vi "MainCondenser.vi"() -> ()   [LabVIEW 2017]
uses:
  <vilib>/Utility/miscctls.llb/LVRowAndColumnTypeDef.ctl
  <vilib>/Utility/sysdir.llb/System Directory Type.ctl
  <vilib>/Utility/config.llb/Read Key (String).vi
  <vilib>/Utility/config.llb/Write Key (String).vi
  <vilib>/Utility/cursorutil.llb/Set Cursor (Icon Pict).vi
  <vilib>/Utility/config.llb/NI_LVConfig.lvlib
panel:
  out "TesterCOM":refnum<visa-resource-name>
  out "CurrentSens":bool
  out "CurrentOut":dbl
  out "Current":string
  out "VISA Current":refnum<visa-resource-name>
  out "TestinExecution":string
  out "FullSpeed2 Current":dbl
  out "FullSpeed1 Current":dbl
  out "String":string
  out "ParamVersion":string
  out "DSP Board S/N":string
  out "POWER Board S/N":string caption="DRIVER Board S/N"
  in  "EventTimeout":i32=100
  out "TestArray":string[](array[string])
  out "Motor Speed RPM Serial":dbl
  out "PN":string
  out "FileName":string
  out "VenableSpeed":u16
  out "TesterVersion":string
  out "ClosePanel":bool=TRUE
  out "UUT SN Report":string
  out "Automation":bool
  out "Test Failed":bool
  out "VenableDirectionResult":bool
  out "VenableResult":bool
  out "ComTestResult":bool=TRUE
  out "UUT SoftwareVer":string
  out "Next SN":i32
  in  "SetSN":bool
  out "Current SN":i32
  out "FullSpeed2 Speed":dbl
  out "FullSpeed2 Current":dbl
  out "FullSpeed1 Current":dbl
  out "FullSpeed1 Speed":dbl
  out "UUT":u8
  out "Tester Status":bool
  out "UUT":string="EBAY"
  in  "Logger Path":path
  in  "Report":bool
  in  "Start":bool
  in  "ATR":string[][](table)=[["Test Communication", "-", "-", "-", "-", ""], ["Set S/N", "-", "-", "-", "-", ""], ["Set Board Number", "-", "-", "-", "-", ""], [" ", "", "", "", "", ""], ["Test Communication", "-", "-", "-", "-", ""], ["Get S/N", "-", "-", "-", "", ""], ["Get Board Number", "-", "-", "-", "", ""], ["Get FW", "-", "-", "-", "", ""], ["Enable Motor", "", "", "", "", ""], ["Small position command", "", "", "", "", ""], ["Measure delta", "", "", "", "", ""], ["Velocity command", "", "", "", "", ""]]
  in  "Settings":bool
  in  "Refresh Button":bool
  out "Serial Status":bool
  in  "VISA Kinetics":refnum<visa-resource-name>="COM6"
  in  "Serial Com":bool
  in  "Help Button":bool
  out "Pannel User Message":string
  in  "Stop Button":bool
  # "Kinetics"
  # "REDLER TECHNOLOGIES LTD"
  # "ver 1.2p"
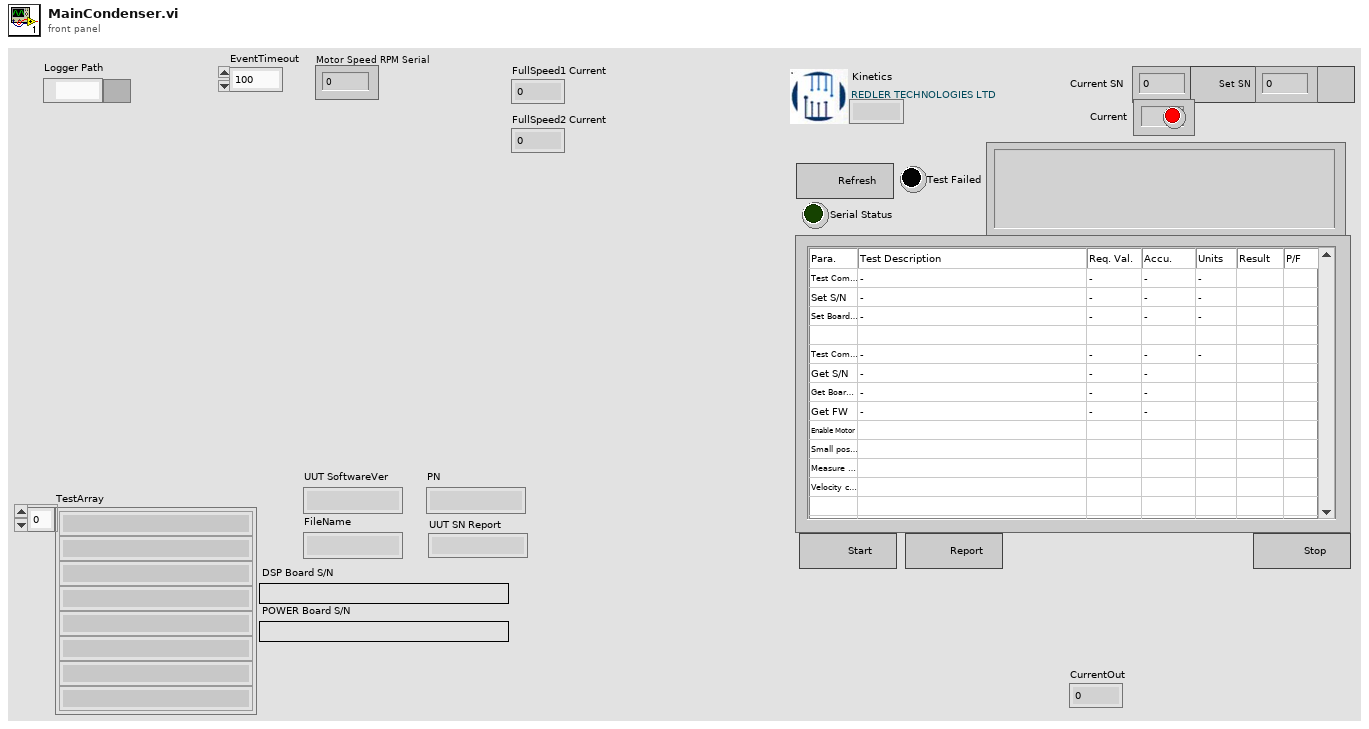
[diagram p1: front panel]
types:
  T1 = cluster{"VISA":refnum<visa-resource-name>, "TestArray":string[]}
  T2 = enum16{"Erase ATR Table", "Stop", "MainProgram", "Initialize"}
  T3 = typedef "NI_LVConfig.lvlib/Config Data RefNum.ctl" = refnum<k1>
  T4 = enum16{"Wait", "Exit", "VC=0", "ReadVC", "VC=1000"}
  T5 = enum16{"Stop", "Result", "FullSpeed2", "MD[1]=1", "FullSpeed1", "MD[1]=0"}
  T6 = enum16{"K15", "K16", "K17", "Venable", "Firmeware", "Fan", "Power", "120C", "110C", "100C", "90C", "80C", "70C", "60C", "50C", "40C", "30C", "25C", "20C", "10C", "0C"}
  T7 = enum8{"Term1", "Term2", "Current", "Fan", "TempCPU"}
  T8 = enum16{"Exit", "Wait", "ReadCurrent", "ReadTemp", "Init"}
  T9 = enum8{"Enabled", "Disabled", "Disabled and Grayed Out"}
  T10 = typedef "LVRowAndColumnTypeDef.ctl" = cluster{"Row":i32, "Column":i32}
  T11 = enum32{"Invalid", "Standard", "Closed", "Hidden", "Minimized", "Maximized"}
  T12 = enum16{"open", "replace", "create", "open or create", "replace or create", "replace or create with confirmation"}
  T13 = typedef "LVPoint32TypeDef.ctl" = cluster{"Horizontal":i32, "Vertical":i32}
  T14 = typedef "System Directory Type.ctl" = i32
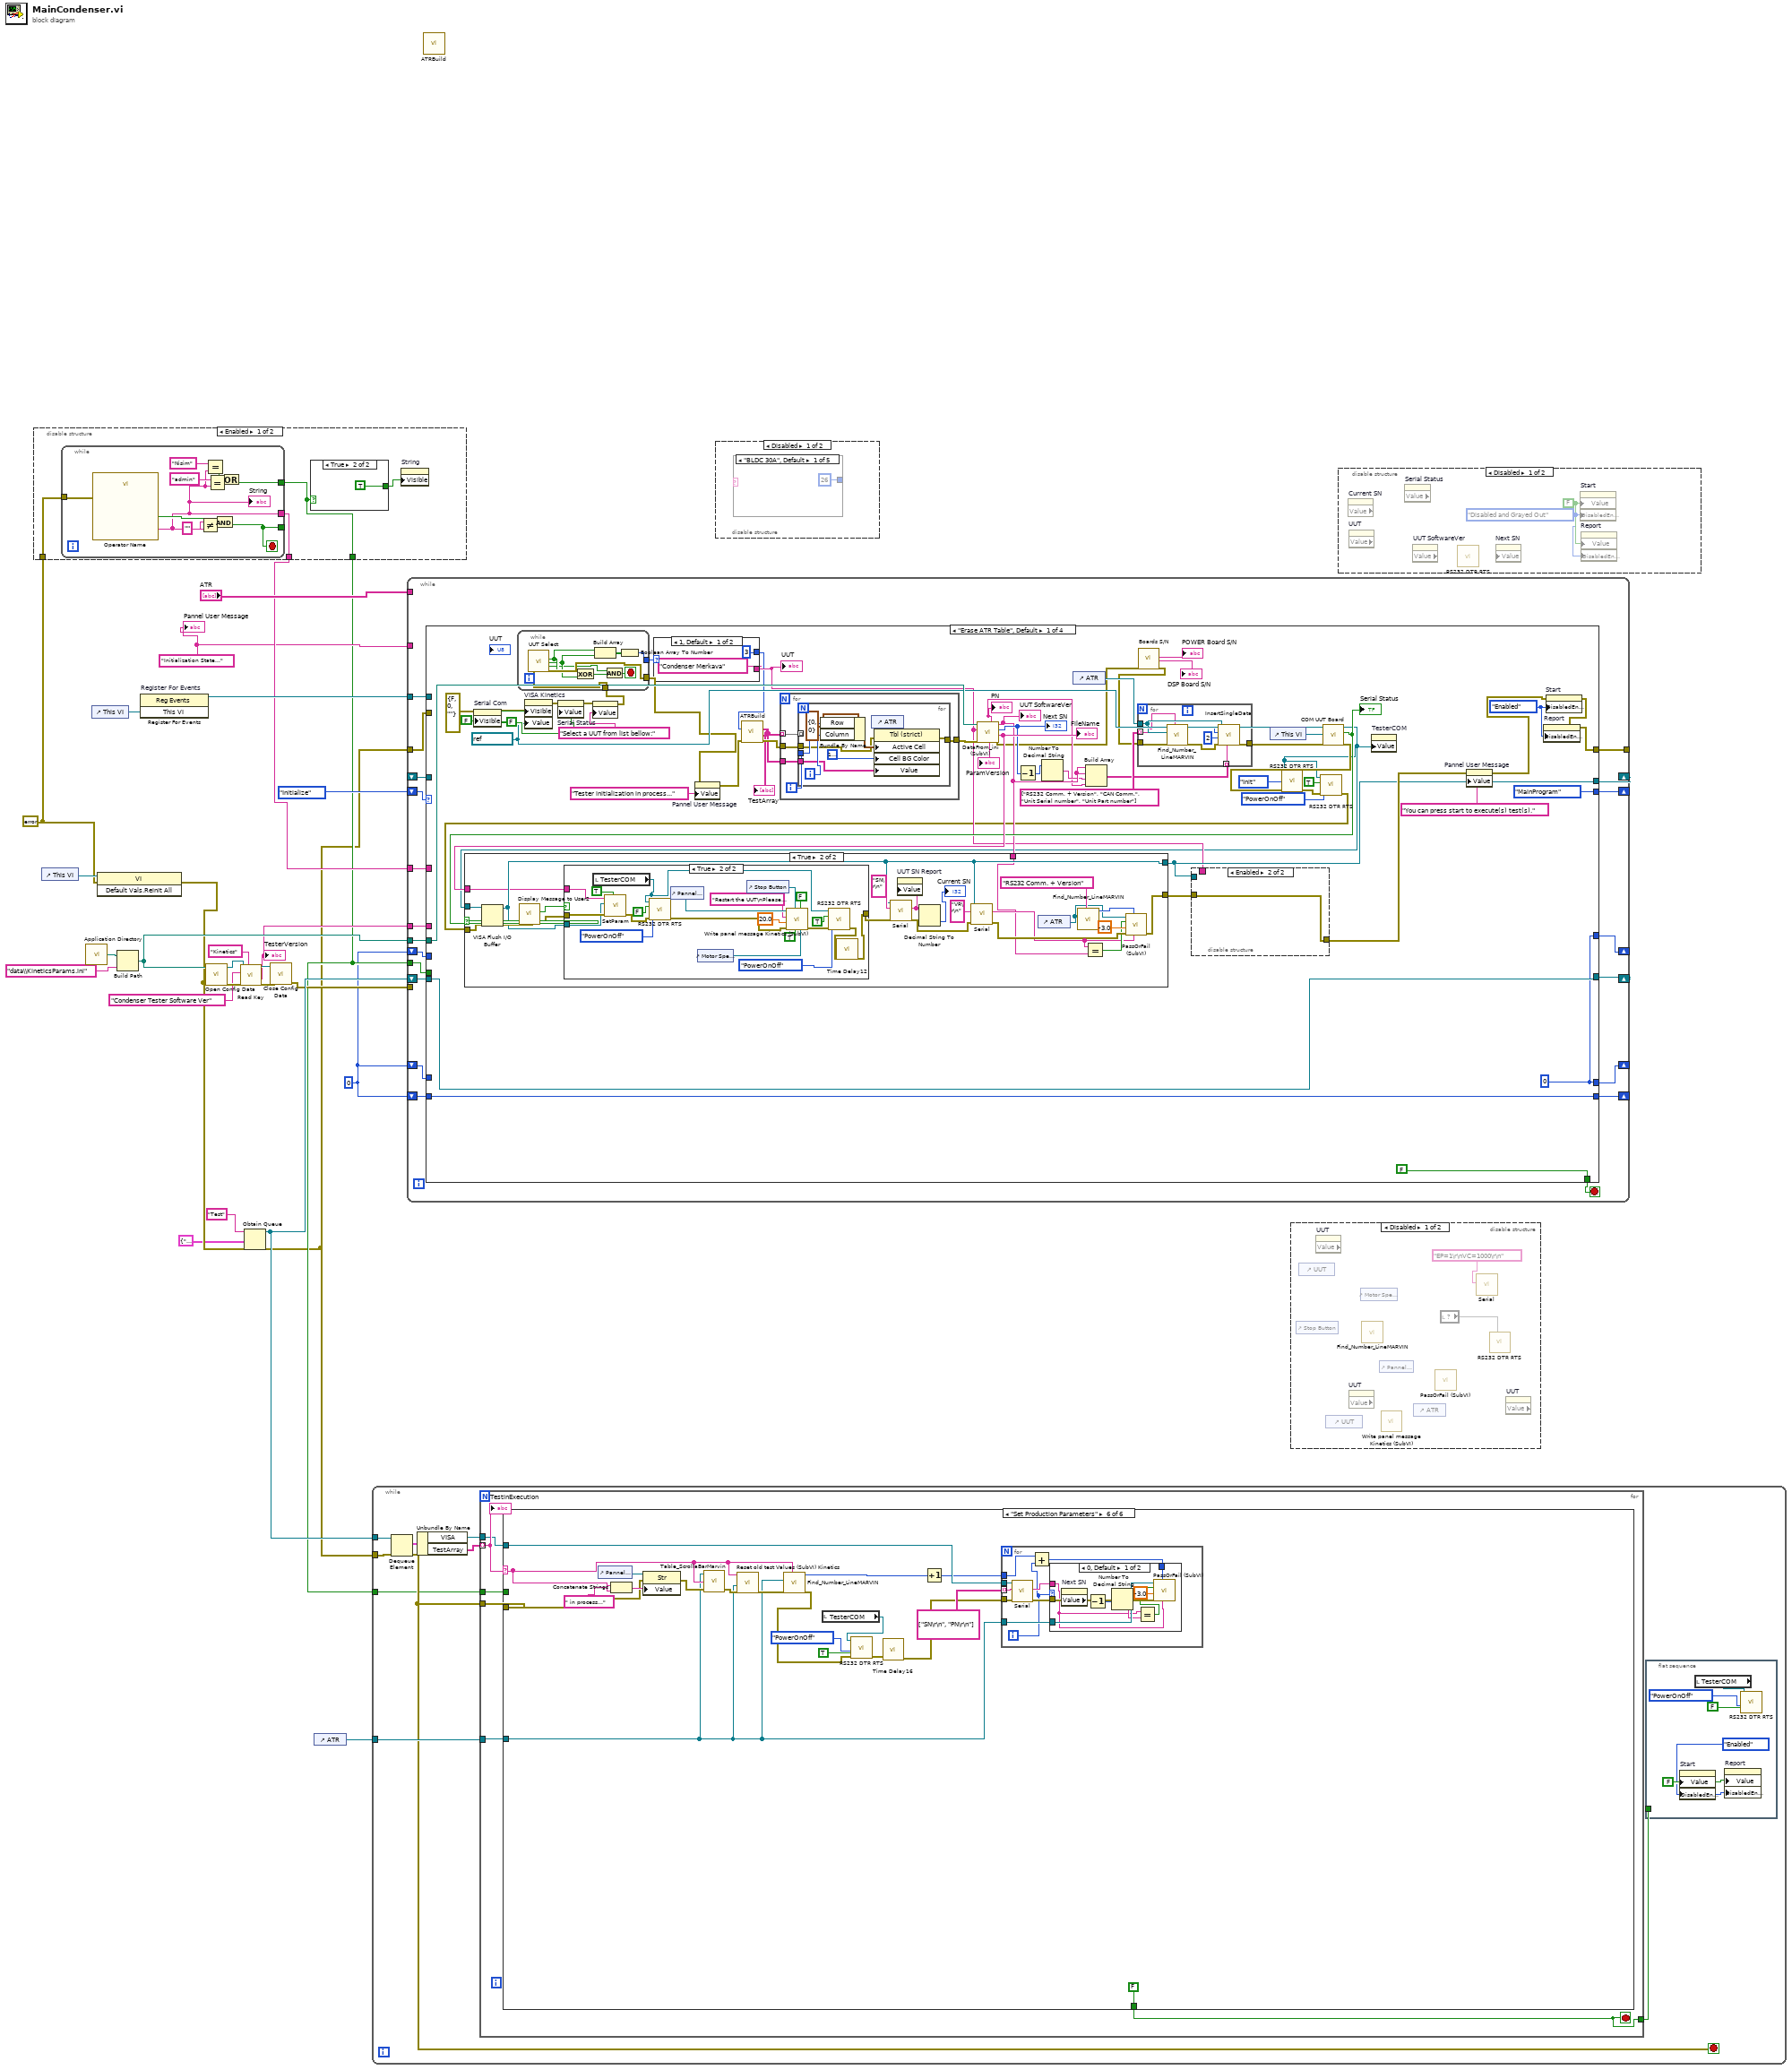
[diagram p0: block diagram]
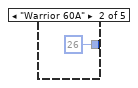
[diagram p2: hidden frame]
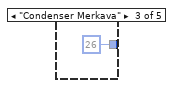
[diagram p3: hidden frame]
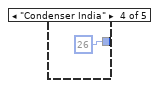
[diagram p4: hidden frame]
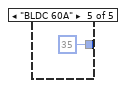
[diagram p5: hidden frame]
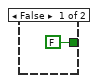
[diagram p7: hidden frame]
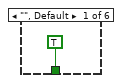
[diagram p11: hidden frame]
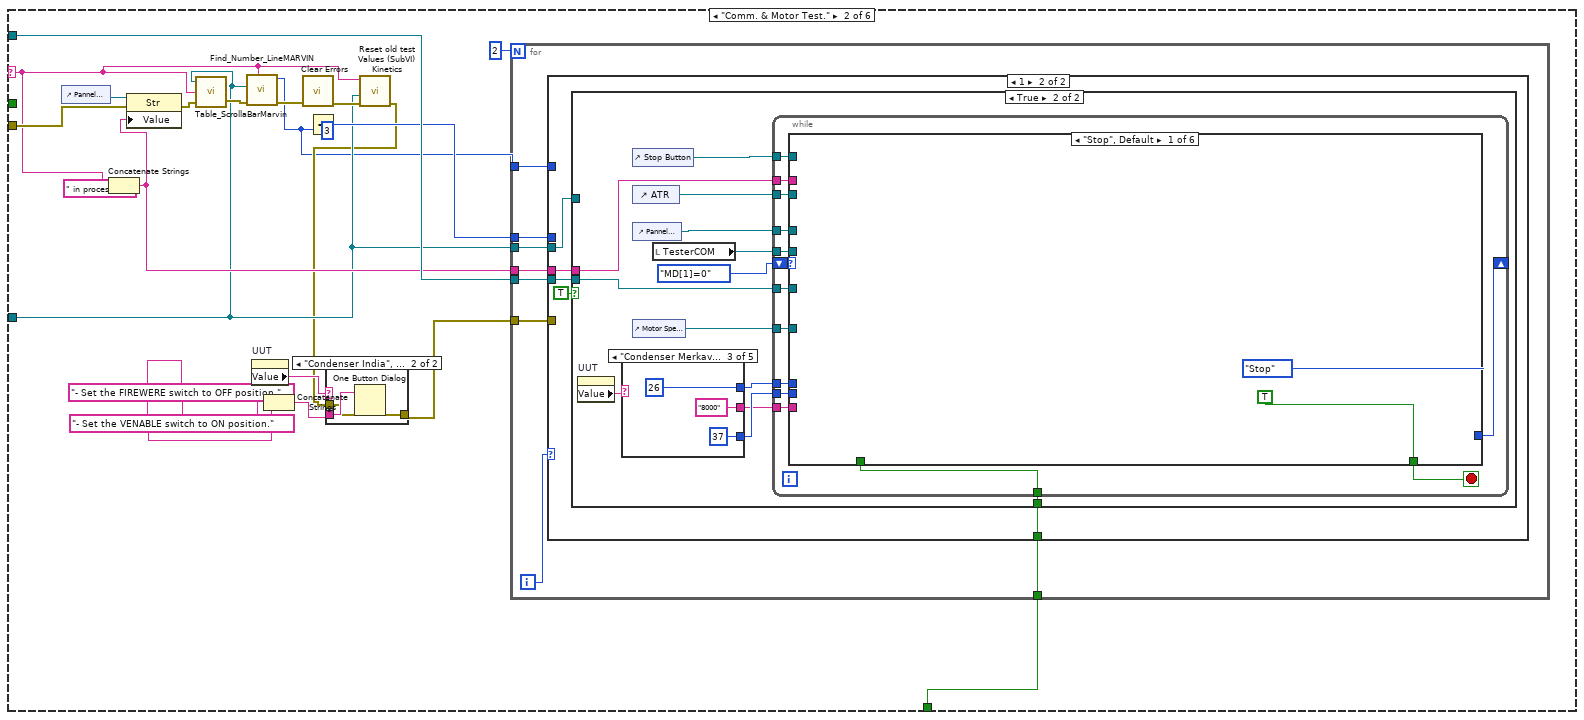
[diagram p12: hidden frame]
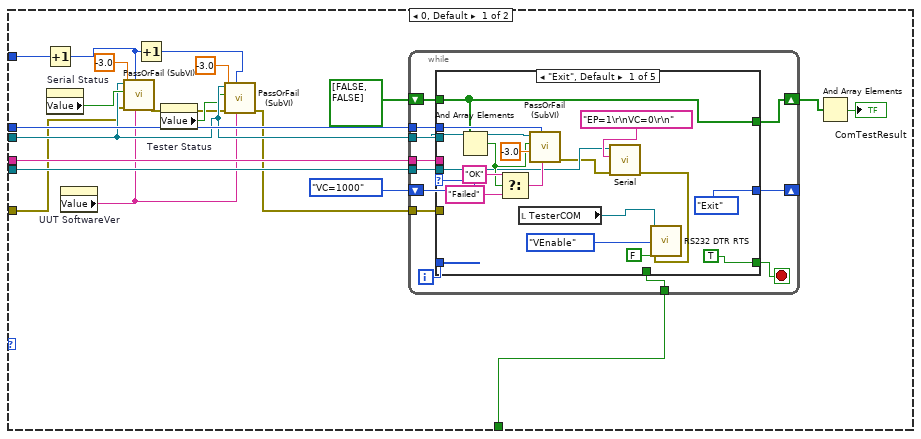
[diagram p13: hidden frame]
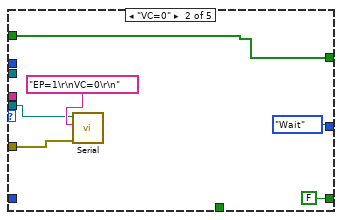
[diagram p14: hidden frame]
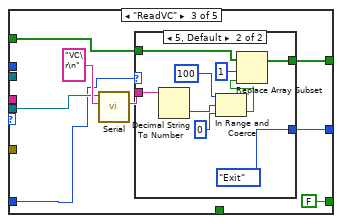
[diagram p15: hidden frame]
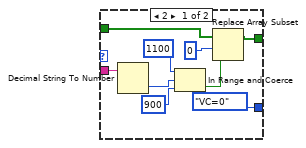
[diagram p16: hidden frame]
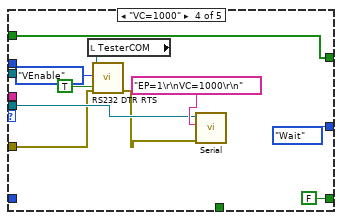
[diagram p17: hidden frame]
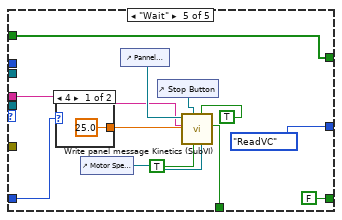
[diagram p18: hidden frame]
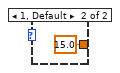
[diagram p19: hidden frame]
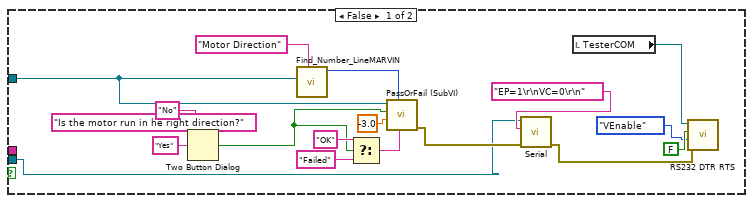
[diagram p20: hidden frame]
diagram:
  w18 = "Initialization State..."
  w3 = 0
  w6 = errorcluster {"status"=FALSE, "code"=0, "source"=""} ("error in (no error)")
  n1 = disable-structure shown="Enabled" {
    disable-tunnel: [w31 _] -> w19
    disable-tunnel: w6 -> [w29 _]
    disable-tunnel: [w28 _] -> w4
    frame Enabled {
      n2 = while {
        tunnel: [w41] -> _
        tunnel: [w34] -> w31
        tunnel: [w38] -> w28
        tunnel: w29 -> [w35]
        stop <- w41 stop-if-true
        n3 = call "Operator Name"("error in (no error)"=w35) -> ("Operator Name"=w34:string, "OK"=w42:bool)  [unwired: 16 in, 1 out]
        "String" <- w34
        n4 = Not Equal?(x=w34, y="") -> (x != y?=w43:bool)
        n5 = Equal?(x="Nisim", y=w34) -> (x = y?=w36:bool)
        n6 = Equal?(x="admin", y=w34) -> (x = y?=w39:bool)
        n7 = And(x=w42, y=w43) -> (x .and. y?=w41:bool)
        n8 = Or(x=w36, y=w39) -> (x .or. y?=w38:bool)
      }
      n9 = case shown="True" w28 {
        tunnel: [FALSE TRUE] -> w30
        frame False {
        }
        frame True {
        }
      }
      n10 = property on="String" class="Str"("Visible"=w30) -> ()  [unwired: 2 in, 2 out]
    }
    frame Disabled {
    }
  }
  n11 = control-ref of="This VI"() -> (w7:refnum<vi>)
  n12 = call <vilib>:"Application Directory.vi"() -> ("Application Directory"=w23:path)
  n13 = control-ref of="This VI"() -> (w21:refnum<vi>)
  n14 = invoke class="VI" method="Default Vals.Reinit All"(reference=w7, error in=w6) -> (error out=w5:errorcluster)  [unwired: 1 in, 2 out]
  n15 = Build Path(base path=w23, name or relative path="data\\KineticsParams.ini") -> (appended path=w10:path)
  n16 = register-events "Register For Events"(w21) -> (reference out=w20:refnum<event-registration>)  [unwired: 2 in, 1 out]
  n17 = call <vilib>:"Open Config Data.vi"("error in (no error)"=w5, "configuration file path"=w10) -> ("error out"=w16:errorcluster, "refnum"=w15:T3)  [unwired: 1 in, 7 out]
  n18 = call-poly <vilib>:"Read Key.vi"("section"="Kinetics", "error in (no error)"=w16, "key"="Condenser Tester Software Ver", "refnum"=w15) -> ("error out"=w13:errorcluster, "value"=w8:string, "refnum out"=w12:T3)  [unwired: 2 in, 3 out]
  "TesterVersion" <- w8
  n19 = Obtain Queue(name (unnamed)="Test", element data type=T1 {"VISA"="COM1", "TestArray"=[]}, error in (no error)=w5) -> (queue out=w25:refnum<queue>, error out=w1:errorcluster)  [unwired: 2 in, 1 out]
  n20 = call <vilib>:"Close Config Data.vi"("error in (no error)"=w13, "refnum"=w12) -> ("error out"=w11:errorcluster)  [unwired: 8 in, 1 out]
  n21 = control-ref of="ATR"() -> (w17:refnum<vi>)
  n22 = while {
    tunnel: w17 -> [w53]
    tunnel: w1 -> [w51]
    tunnel: w25 -> [w52]
    tunnel: w4 -> [w46]
    stop <- w48 stop-if-true
    n23 = Dequeue Element(queue=w52, error in (no error)=w51) -> (element=w50:T1, error out=w48:errorcluster)  [unwired: 1 in, 2 out]
    n24 = Unbundle By Name(w50) -> ("VISA"=w49:refnum<visa-resource-name>, "TestArray"=w45:string[])
    n25 = for {
      tunnel: w45 -> [w63] mode=indexing
      tunnel: w49 -> [w61]
      tunnel: w53 -> [w60]
      tunnel: w48 -> [w64]
      tunnel: [w59] -> w47
      tunnel: w46 -> [w62]
      stop <- w59 stop-if-true
      n26 = case shown="\"Set Production Parameters\"" w63 {
        selector: w63 -> [_ w82 w503 w964 w1087 w1211]
        tunnel: w60 -> [_ w75 _ _ w1095 w1209]
        tunnel: w64 -> [_ w85 _ _ w1100 w1213]
        tunnel: w62 -> [_ _ _ _ _ _]
        tunnel: w61 -> [_ w78 w502 w963 w1088 w1210]
        tunnel: [TRUE ("Stopped") w70 w501 w953 w1086 FALSE ("Stopped")] -> w59
        frame "", Default {
        }
        frame "Comm. & Motor Test." {
          n27 = control-ref of="Pannel User Message"() -> (w86:refnum<vi>)
          n28 = Concatenate Strings(w82, " in process..." ("string")) -> (w77:string)
          n29 = property class="Str"(reference=w86, error in=w85, "Value"=w77) -> (error out=w84:errorcluster)  [unwired: 1 out]
          n30 = call "Table_ScrollaBarMarvin.vi"("error in"=w84, "Line to focus"=w82, "reference in"=w75) -> ("error out"=w81:errorcluster)  [unwired: 2 out]
          n31 = call "Find_Number_LineMARVIN.vi"("Test Paragraph"=w82, "error in"=w81, "TableIn"=w75) -> ("error out"=w87:errorcluster, "Line number"=w66:i32)  [unwired: 2 in, 2 out]
          n32 = property on="UUT" class="Str"() -> ("Value"=w74:string)  [unwired: 2 in, 2 out]
          n33 = Concatenate Strings("- Set the FIREWERE switch to OFF position." ("Screen Line"), "- Set the VENABLE switch to ON position." ("Screen Line")) -> (w71:string)
          n34 = call <vilib>:"Clear Errors.vi"("error in (no error)"=w87) -> ("error out"=w80:errorcluster)  [unwired: 5 in, 1 out]
          n35 = Add(x=3, y=w66) -> (x+y=w76:i32)
          n36 = call "Reset old test Values (SubVI) Kinetics.vi"("error in"=w80, "Atr in"=w75, "Test Paragraph"=w82) -> ("error out"=w69:errorcluster)  [unwired: 6 in, 2 out]
          n37 = case shown="\"Condenser India\", \"Condenser Merkava\"" w74 {
            tunnel: w71 -> [_ w500]
            tunnel: w69 -> [w498 w499]
            tunnel: [w498 w499] -> w68
            frame "False", Default {
            }
            frame "Condenser India", "Condenser Merkava" {
              n38 = One Button Dialog(message=w500) -> ()  [unwired: 1 in, 1 out]
            }
          }
          n39 = for {
            N: 2 -> [_]
            tunnel: w78 -> [w95]
            tunnel: w77 -> [w94]
            tunnel: w76 -> [w93]
            tunnel: w75 -> [w92]
            tunnel: [w91] -> w70
            tunnel: w68 -> [w90]
            tunnel: w66 -> [w88]
            i -> [w89]
            n40 = case shown="1" w89 {
              tunnel: w95 -> [w113 w204]
              tunnel: w94 -> [w112 w203]
              tunnel: w93 -> [w110 _]
              tunnel: w92 -> [w103 w201]
              tunnel: [w108 w205] -> w91
              tunnel: w90 -> [w99 _]
              tunnel: w88 -> [w105 _]
              frame 0, Default {
                n41 = Increment(x=w105) -> (x+1=w98:i32)
                n42 = property on="Serial Status" class="Bool (strict)"() -> ("Value"=w107:bool)  [unwired: 2 in, 2 out]
                n43 = property on="UUT SoftwareVer" class="Str"() -> ("Value"=w96:string)  [unwired: 2 in, 2 out]
                n44 = call "PassOrFail (SubVI).vi"("String Res"=w96, "index (row)"=w98, "error in (no error)"=w99, "Data in"=-3.0, "Pass?Fail"=w107, "Table in"=w103) -> ("error out"=w101:errorcluster)  [unwired: 5 in]
                n45 = Increment(x=w98) -> (x+1=w97:i32)
                n46 = property on="Tester Status" class="Bool (strict)"() -> ("Value"=w102:bool)  [unwired: 2 in, 2 out]
                n47 = call "PassOrFail (SubVI).vi"("String Res"=w96, "index (row)"=w97, "error in (no error)"=w101, "Data in"=-3.0, "Pass?Fail"=w102, "Table in"=w103) -> ("error out"=w100:errorcluster)  [unwired: 5 in]
                n48 = while {
                  shift-right: [w124] -> _
                  shift-left: T4."VC=1000" -> [w127]
                  tunnel: w100 -> [w126]
                  tunnel: w113 -> [w125]
                  tunnel: w112 -> [w123]
                  shift-right: [w120] -> w109
                  shift-left: bool[] [FALSE, FALSE] -> [w121]
                  tunnel: w110 -> [w119]
                  tunnel: w103 -> [w118]
                  tunnel: [w116] -> w108
                  i -> [w122]
                  stop <- w117 stop-if-true
                  n49 = case shown="\"Exit\", Default" w127 {
                    tunnel: w126 -> [_ w150 _ w182 _]
                    tunnel: w125 -> [w132 w148 w157 w185 _]
                    tunnel: [T4."Exit" T4."Wait" w154 T4."Wait" T4."ReadVC"] -> w124
                    tunnel: w123 -> [_ _ _ _ w193]
                    tunnel: [TRUE FALSE FALSE FALSE FALSE] -> w117
                    tunnel: w122 -> [_ _ w155 _ w188]
                    tunnel: w121 -> [w131 w145 w153 w183 w190]
                    tunnel: [w131 w145 w152 w183 w190] -> w120
                    tunnel: w119 -> [w138 _ _ _ _]
                    tunnel: w118 -> [w140 _ _ _ _]
                    tunnel: [_ _ _ _ w187] -> w116
                    frame "Exit", Default {
                      n50 = And Array Elements(Boolean array=w131) -> (logical AND=w135:bool)
                      n51 = Select(t="OK", s=w135, f="Failed") -> (s? t:f=w139:string)
                      n52 = local read "TesterCOM"() -> (w128:refnum<visa-resource-name>)
                      n53 = call "PassOrFail (SubVI).vi"("String Res"=w139, "index (row)"=w138, "Data in"=-3.0, "Pass?Fail"=w135, "Table in"=w140) -> ("error out"=w130:errorcluster)  [unwired: 6 in]
                      n54 = call "Serial.vi"("error in (no error)"=w130, "write buffer"="EP=1\r\nVC=0\r\n", "VISA resource name"=w132) -> ("error out"=w133:errorcluster)  [unwired: 7 in, 1 out]
                      n55 = call "RS232 DTR RTS.vi"("error in (no error)"=w133, "Func"=enum16{"Init", "VEnable", "PowerOnOff"}."VEnable", "On/Off"=FALSE, "TesterCOM in"=w128) -> ()  [unwired: 7 in, 1 out]
                    }
                    frame "VC=0" {
                      n56 = call "Serial.vi"("error in (no error)"=w150, "write buffer"="EP=1\r\nVC=0\r\n", "VISA resource name"=w148) -> ()  [unwired: 7 in, 2 out]
                    }
                    frame "ReadVC" {
                      n57 = call "Serial.vi"("write buffer"="VC\r\n", "VISA resource name"=w157) -> ("read buffer"=w156:string)  [unwired: 8 in, 1 out]
                      n58 = case shown="5, Default" w155 {
                        tunnel: w156 -> [w166 w172]
                        tunnel: [T4."VC=0" T4."Exit"] -> w154
                        tunnel: w153 -> [w161 w171]
                        tunnel: [w159 w168] -> w152
                        frame 2 {
                          n59 = Decimal String To Number(string=w166) -> (number=w165:i32)  [unwired: 2 in, 1 out]
                          n60 = In Range and Coerce(upper limit=1100, x=w165, lower limit=900) -> (In Range?=w160:bool)  [unwired: 1 out]
                          n61 = Replace Array Subset(array=w161, new element=w160, index=0) -> (w159:bool[])
                        }
                        frame 5, Default {
                          n62 = Decimal String To Number(string=w172) -> (number=w175:i32)  [unwired: 2 in, 1 out]
                          n63 = In Range and Coerce(upper limit=100, x=w175, lower limit=0) -> (In Range?=w169:bool)  [unwired: 1 out]
                          n64 = Replace Array Subset(array=w171, new element=w169, index=1) -> (w168:bool[])
                        }
                      }
                    }
                    frame "VC=1000" {
                      n65 = local read "TesterCOM"() -> (w177:refnum<visa-resource-name>)
                      n66 = call "RS232 DTR RTS.vi"("error in (no error)"=w182, "Func"=enum16{"Init", "VEnable", "PowerOnOff"}."VEnable", "On/Off"=TRUE, "TesterCOM in"=w177) -> ("error out"=w181:errorcluster)  [unwired: 7 in]
                      n67 = call "Serial.vi"("error in (no error)"=w181, "write buffer"="EP=1\r\nVC=1000\r\n", "VISA resource name"=w185) -> ()  [unwired: 7 in, 2 out]
                    }
                    frame "Wait" {
                      n68 = case shown="4" w188 {
                        tunnel: [25.0 ("Time to wait") 15.0 ("Time to wait")] -> w194
                        frame 4 {
                        }
                        frame 1, Default {
                        }
                      }
                      n69 = control-ref of="Motor Speed RPM Serial"() -> (w198:refnum<vi>)
                      n70 = control-ref of="Pannel User Message"() -> (w197:refnum<vi>)
                      n71 = control-ref of="Stop Button"() -> (w192:refnum<vi>)
                      n72 = call "Write panel message Kinetics (SubVI).vi"(4:"rpm"=w198, 5:"rpm"=TRUE ("rpm"), "PrintTime"=TRUE, "Stop"=w192, "Time to wait"=w194, "Strin"=w193, "String in"=w197) -> ("Stopped"=w187:bool)  [unwired: 3 in, 1 out]
                    }
                  }
                }
                n73 = And Array Elements(Boolean array=w109) -> (logical AND=→"ComTestResult":bool)
              }
              frame 1 {
                n74 = case shown="True" TRUE {
                  tunnel: [_ w227] -> w205
                  tunnel: w204 -> [w208 w226]
                  tunnel: w203 -> [_ w224]
                  tunnel: w201 -> [w213 _]
                  frame False {
                    n75 = Two Button Dialog(message="Is the motor run in he right direction?", 1:"No" ("F button name (\"Cancel\")"), 2:"Yes" ("T button name (\"OK\")")) -> (T button?=w209:bool)
                    n76 = call "Find_Number_LineMARVIN.vi"("Test Paragraph"="Motor Direction", "TableIn"=w213) -> ("Line number"=w223:i32)  [unwired: 3 in, 3 out]
                    n77 = Select(t="OK", s=w209, f="Failed") -> (s? t:f=w222:string)
                    n78 = call "PassOrFail (SubVI).vi"("String Res"=w222, "index (row)"=w223, "Data in"=-3.0, "Pass?Fail"=w209, "Table in"=w213) -> ("error out"=w220:errorcluster)  [unwired: 6 in]
                    n79 = call "Serial.vi"("error in (no error)"=w220, "write buffer"="EP=1\r\nVC=0\r\n", "VISA resource name"=w208) -> ("error out"=w221:errorcluster)  [unwired: 7 in, 1 out]
                    n80 = local read "TesterCOM"() -> (w207:refnum<visa-resource-name>)
                    n81 = call "RS232 DTR RTS.vi"("error in (no error)"=w221, "Func"=enum16{"Init", "VEnable", "PowerOnOff"}."VEnable", "On/Off"=FALSE, "TesterCOM in"=w207) -> ()  [unwired: 7 in, 1 out]
                  }
                  frame True {
                    n82 = property on="UUT" class="Str"() -> ("Value"=w229:string)  [unwired: 2 in, 2 out]
                    n83 = case shown="\"Condenser Merkava\"" w229 {
                      tunnel: [26 26 26 26 40] -> w230
                      tunnel: [_ _ 37 37 56] -> w231
                      tunnel: [_ _ "8000" "8000" "10800"] -> w225
                      frame "BLDC 30A", Default {
                      }
                      frame "Warrior 60A" {
                      }
                      frame "Condenser Merkava" {
                      }
                      frame "Condenser India" {
                      }
                      frame "BLDC 60A" {
                      }
                    }
                    n84 = control-ref of="Stop Button"() -> (w232:refnum<vi>)
                    n85 = control-ref of="ATR"() -> (w236:refnum<vi>)
                    n86 = control-ref of="Pannel User Message"() -> (w233:refnum<vi>)
                    n87 = control-ref of="Motor Speed RPM Serial"() -> (w234:refnum<vi>)
                    n88 = local read "TesterCOM"() -> (w235:refnum<visa-resource-name>)
                    n89 = while {
                      shift-right: [w249] -> _
                      shift-left: T5."MD[1]=0" -> [w250]
                      tunnel: w232 -> [w248]
                      tunnel: w233 -> [w247]
                      tunnel: w234 -> [w246]
                      tunnel: w235 -> [w245]
                      tunnel: w230 -> [w244]
                      tunnel: w231 -> [w243]
                      tunnel: w236 -> [w242]
                      tunnel: [w237] -> w227
                      tunnel: w226 -> [w240]
                      tunnel: w225 -> [w239]
                      tunnel: w224 -> [w238]
                      stop <- w241 stop-if-true
                      n90 = case shown="\"Stop\", Default" w250 {
                        tunnel: [T5."Stop" T5."Stop" w316 w389 w413 w486] -> w249
                        tunnel: [TRUE w266 FALSE FALSE FALSE FALSE] -> w241
                        tunnel: w248 -> [_ w258 w301 w369 w399 w466]
                        tunnel: w247 -> [_ w257 w302 w370 w400 w467]
                        tunnel: w246 -> [_ w256 w303 w364 w402 w461]
                        tunnel: w245 -> [_ w254 w306 w348 _ w445]
                        tunnel: w244 -> [_ _ _ _ w401 _]
                        tunnel: w243 -> [_ _ w300 _ _ _]
                        tunnel: w242 -> [_ w268 _ _ _ _]
                        tunnel: w240 -> [_ w262 w296 w353 w397 w458]
                        tunnel: w239 -> [_ _ w295 _ w394 _]
                        tunnel: w238 -> [_ _ w293 w361 w392 w457]
                        tunnel: [_ _ w292 w354 w391 w450] -> w237
                        frame "Stop", Default {
                        }
                        frame "Result" {
                          n91 = property on="FullSpeed2 Current" class="DigNum (strict)"() -> ("Value"=w273:dbl)  [unwired: 2 in, 2 out]
                          n92 = property on="FullSpeed1 Current" class="DigNum (strict)"() -> ("Value"=w272:dbl)  [unwired: 2 in, 2 out]
                          n93 = Subtract(x=w273, y=w272) -> (x-y=w280:dbl)
                          n94 = call "Find_Number_LineMARVIN.vi"("Test Paragraph"="Motor Direction", "TableIn"=w268) -> ("Line number"=w277:i32)  [unwired: 3 in, 3 out]
                          n95 = Absolute Value(x=w280) -> (abs(x)=w275:dbl)
                          n96 = Greater Or Equal?(x=w275, y=u32 5) -> (x >= y?=w267:bool)
                          n97 = Select(t="OK", s=w267, f="Failed") -> (s? t:f=w269:string)
                          n98 = call "PassOrFail (SubVI).vi"("String Res"=w269, "index (row)"=w277, "Data in"=-3.0, "Pass?Fail"=w267, "Table in"=w268) -> ("error out"=w261:errorcluster)  [unwired: 6 in]
                          n99 = call "Serial.vi"("error in (no error)"=w261, "write buffer"="EP=1\r\nVC=0\r\n", "VISA resource name"=w262) -> ("error out"=w265:errorcluster)  [unwired: 7 in, 1 out]
                          n100 = call "RS232 DTR RTS.vi"("error in (no error)"=w265, "Func"=enum16{"Init", "VEnable", "PowerOnOff"}."VEnable", "On/Off"=FALSE, "TesterCOM in"=w254) -> ("error out"=w259:errorcluster)  [unwired: 7 in]
                          n101 = while {
                            tunnel: w259 -> [w288]
                            tunnel: w258 -> [w287]
                            tunnel: w257 -> [w286]
                            tunnel: w256 -> [w284]
                            tunnel: "Please wait untill RPM = 0." -> [w285]
                            stop <- w281 stop-if-true
                            n102 = property class="DigNum (strict)"(reference=w284) -> ("Value"=w283:dbl)  [unwired: 1 in, 2 out]
                            n103 = call "Write panel message Kinetics (SubVI).vi"(4:"rpm"=w284, 5:"rpm"=TRUE ("rpm"), "PrintTime"=FALSE, "Stop"=w287, "error in (no error)"=w288, "Time to wait"=0.2, "Strin"=w285, "String in"=w286) -> ()  [unwired: 2 in, 2 out]
                            n104 = Less Or Equal?(x=w283, y=50.0) -> (x <= y?=w281:bool)
                          }
                          n105 = Not(x=TRUE) -> (.not. x?=w266:bool)
                        }
                        frame "FullSpeed2" {
                          n106 = Search and Replace String(input string="EP=1\r\nVC=0\r\n" ("write buffer"), search string="0", replace string=w295) -> (result string=w299:string)  [unwired: 5 in, 3 out]
                          n107 = call "Serial.vi"("write buffer"=w299, "VISA resource name"=w296) -> ("error out"=w294:errorcluster)  [unwired: 8 in, 1 out]
                          n108 = Concatenate Strings(w293, "\nFull speed operation " ("string")) -> (w310:string)
                          n109 = call "Write panel message Kinetics (SubVI).vi"(4:"rpm"=w303, 5:"rpm"=TRUE ("rpm"), "PrintTime"=TRUE, "Stop"=w301, "error in (no error)"=w294, "Time to wait"=45.0, "Strin"=w310, "String in"=w302) -> ("error out"=w313:errorcluster, "Stopped"=w305:bool)  [unwired: 2 in]
                          n110 = flat-sequence {
                            tunnel: w313 -> [w320]
                            tunnel: [w320] -> w312
                            tunnel: [w319] -> w311
                            frame #0 {
                              n111 = call <vilib>:"High Resolution Relative Seconds.vi"() -> ("relative seconds"=w319:dbl)
                            }
                          }
                          n112 = while {
                            tunnel: w312 -> [_]
                            tunnel: [w342] -> _
                            tunnel: w300 -> [w346]
                            tunnel: w311 -> [w344]
                            tunnel: w310 -> [w340]
                            tunnel: w303 -> [w333]
                            tunnel: w306 -> [_]
                            tunnel: w305 -> [w337]
                            tunnel: [w325] -> w304
                            tunnel: w302 -> [w336]
                            tunnel: w301 -> [w335]
                            tunnel: [w328] -> w292
                            stop <- w347 stop-if-true
                            n113 = call <vilib>:"High Resolution Relative Seconds.vi"() -> ("relative seconds"=w345:dbl)
                            n114 = local read "CurrentOut"() -> (w327:dbl)
                            n115 = property class="DigNum (strict)"(reference=w333) -> ("Value"=w332:dbl)  [unwired: 1 in, 2 out]
                            n116 = Subtract(x=w345, y=w344) -> (x-y=w323:dbl)
                            n117 = Greater Or Equal?(x=w323, y=60.0) -> (x >= y?=w324:bool)
                            n118 = To Double Precision Float(number=w327) -> (double precision float=w326:dbl)
                            "FullSpeed2 Current" <- w326
                            n119 = Greater Or Equal?(x=w326, y=w346) -> (x >= y?=w334:bool)
                            n120 = Greater Or Equal?(x=w323, y=15.0) -> (x >= y?=w321:bool)
                            n121 = Greater Or Equal?(x=w332, y=7200.0) -> (x >= y?=w329:bool)
                            n122 = And(x=w334, y=w329) -> (x .and. y?=w330:bool)
                            n123 = call "Write panel message Kinetics (SubVI).vi"(4:"rpm"=w333, 5:"rpm"=TRUE ("rpm"), "PrintTime"=FALSE, "Stop"=w335, "Time to wait"=0.2, "Strin"=w340, "String in"=w336) -> ("error out"=w342:errorcluster, "Stopped"=w328:bool)  [unwired: 3 in]
                            n124 = Compound Arithmetic op=OR(w321, w328, w324) -> (w325:bool)
                            n125 = call "Display Message to User4"("Enable"=w321) -> ()  [unwired: 9 in, 2 out]
                            n126 = Compound Arithmetic op=OR(w321, w328, w337, w324, w330) -> (w347:bool)
                          }
                          n127 = Select(t=T5."Stop", s=w304, f=T5."Result") -> (s? t:f=w316:T5)
                        }
                        frame "MD[1]=1" {
                          n128 = call "RS232 DTR RTS.vi"("Func"=enum16{"Init", "VEnable", "PowerOnOff"}."VEnable", "On/Off"=FALSE, "TesterCOM in"=w348) -> ("error out"=w377:errorcluster)  [unwired: 8 in]
                          n129 = Concatenate Strings(w361, "\nSet Parameters MD[1]=1" ("Strin")) -> (w371:string)
                          n130 = call "Write panel message Kinetics (SubVI).vi"(4:"rpm"=w364, 5:"rpm"=FALSE ("rpm"), "PrintTime"=FALSE, "Stop"=w369, "error in (no error)"=w377, "Time to wait"=30.0, "Strin"=w371, "String in"=w370) -> ("error out"=w376:errorcluster, "Stopped"=w355:bool)  [unwired: 2 in]
                          n131 = call "Serial.vi"("error in (no error)"=w376, "write buffer"="EP=1\r\nVC=0\r\nMD[1]=1\r\n", "VISA resource name"=w353) -> ("error out"=w374:errorcluster)  [unwired: 7 in, 1 out]
                          n132 = call "RS232 DTR RTS.vi"("error in (no error)"=w374, "Func"=enum16{"Init", "VEnable", "PowerOnOff"}."PowerOnOff", "On/Off"=FALSE, "TesterCOM in"=w348) -> ("error out"=w373:errorcluster)  [unwired: 7 in]
                          n133 = call "Write panel message Kinetics (SubVI).vi"(4:"rpm"=w364, 5:"rpm"=FALSE ("rpm"), "PrintTime"=TRUE, "Stop"=w369, "error in (no error)"=w373, "Time to wait"=25.0, "Strin"=w371, "String in"=w370) -> ("error out"=w358:errorcluster, "Stopped"=w356:bool)  [unwired: 2 in]
                          n134 = call "RS232 DTR RTS.vi"("error in (no error)"=w358, "Func"=enum16{"Init", "VEnable", "PowerOnOff"}."PowerOnOff", "On/Off"=TRUE, "TesterCOM in"=w348) -> ("error out"=w359:errorcluster)  [unwired: 7 in]
                          n135 = call "RS232 DTR RTS.vi"("error in (no error)"=w359, "Func"=enum16{"Init", "VEnable", "PowerOnOff"}."VEnable", "On/Off"=TRUE, "TesterCOM in"=w348) -> ("error out"=w366:errorcluster)  [unwired: 7 in]
                          n136 = call "Write panel message Kinetics (SubVI).vi"(4:"rpm"=w364, 5:"rpm"=FALSE ("rpm"), "PrintTime"=TRUE, "Stop"=w369, "error in (no error)"=w366, "Time to wait"=3.0, "Strin"=w371, "String in"=w370) -> ("Stopped"=w357:bool)  [unwired: 2 in, 1 out]
                          n137 = Compound Arithmetic op=OR(w357, w356, w355) -> (w354:bool)
                          n138 = Compound Arithmetic op=OR(w357, w356, w355) -> (w363:bool)
                          n139 = Select(t=T5."Stop", s=w363, f=T5."FullSpeed2") -> (s? t:f=w389:T5)
                        }
                        frame "FullSpeed1" {
                          n140 = Search and Replace String(input string="EP=1\r\nVC=0\r\n" ("write buffer"), search string="0", replace string=w394) -> (result string=w393:string)  [unwired: 5 in, 3 out]
                          n141 = call "Serial.vi"("write buffer"=w393, "VISA resource name"=w397) -> ("error out"=w398:errorcluster)  [unwired: 8 in, 1 out]
                          n142 = Concatenate Strings(w392, "\nFull speed operation " ("string")) -> (w407:string)
                          n143 = call "Write panel message Kinetics (SubVI).vi"(4:"rpm"=w402, 5:"rpm"=TRUE ("rpm"), "PrintTime"=TRUE, "Stop"=w399, "error in (no error)"=w398, "Time to wait"=45.0, "Strin"=w407, "String in"=w400) -> ("error out"=w410:errorcluster, "Stopped"=w403:bool)  [unwired: 2 in]
                          n144 = flat-sequence {
                            tunnel: w410 -> [w417]
                            tunnel: [w417] -> w409
                            tunnel: [w416] -> w408
                            frame #0 {
                              n145 = call <vilib>:"High Resolution Relative Seconds.vi"() -> ("relative seconds"=w416:dbl)
                            }
                          }
                          n146 = while {
                            tunnel: w409 -> [_]
                            tunnel: [w439] -> _
                            tunnel: w401 -> [w443]
                            tunnel: w408 -> [w441]
                            tunnel: w407 -> [w437]
                            tunnel: w402 -> [w428]
                            tunnel: w403 -> [w433]
                            tunnel: [w422] -> w390
                            tunnel: w400 -> [w432]
                            tunnel: w399 -> [w431]
                            tunnel: [w424] -> w391
                            stop <- w444 stop-if-true
                            n147 = call <vilib>:"High Resolution Relative Seconds.vi"() -> ("relative seconds"=w442:dbl)
                            n148 = local read "CurrentOut"() -> (w423:dbl)
                            n149 = property class="DigNum (strict)"(reference=w428) -> ("Value"=w427:dbl)  [unwired: 1 in, 2 out]
                            n150 = Subtract(x=w442, y=w441) -> (x-y=w420:dbl)
                            n151 = Greater Or Equal?(x=w420, y=60.0) -> (x >= y?=w421:bool)
                            n152 = To Double Precision Float(number=w423) -> (double precision float=→"FullSpeed1 Current":dbl)
                            n153 = Greater Or Equal?(x=w423, y=w443) -> (x >= y?=w430:bool)
                            n154 = Greater Or Equal?(x=w420, y=15.0) -> (x >= y?=w418:bool)
                            n155 = Greater Or Equal?(x=w427, y=7800.0) -> (x >= y?=w425:bool)
                            n156 = And(x=w425, y=w430) -> (x .and. y?=w429:bool)
                            n157 = call "Write panel message Kinetics (SubVI).vi"(4:"rpm"=w428, 5:"rpm"=TRUE ("rpm"), "PrintTime"=FALSE, "Stop"=w431, "Time to wait"=0.2, "Strin"=w437, "String in"=w432) -> ("error out"=w439:errorcluster, "Stopped"=w424:bool)  [unwired: 3 in]
                            n158 = call "Display Message to User6"("Enable"=w418) -> ()  [unwired: 9 in, 2 out]
                            n159 = Compound Arithmetic op=OR(w418, w424, w421) -> (w422:bool)
                            n160 = Compound Arithmetic op=OR(w418, w424, w433, w421, w429) -> (w444:bool)
                          }
                          n161 = Select(t=T5."Stop", s=w390, f=T5."MD[1]=1") -> (s? t:f=w413:T5)
                        }
                        frame "MD[1]=0" {
                          n162 = call "RS232 DTR RTS.vi"("Func"=enum16{"Init", "VEnable", "PowerOnOff"}."VEnable", "On/Off"=FALSE, "TesterCOM in"=w445) -> ("error out"=w474:errorcluster)  [unwired: 8 in]
                          n163 = Concatenate Strings(w457, "\nSet Parameters MD[1]=0" ("Strin")) -> (w468:string)
                          n164 = call "Write panel message Kinetics (SubVI).vi"(4:"rpm"=w461, 5:"rpm"=FALSE ("rpm"), "PrintTime"=FALSE, "Stop"=w466, "error in (no error)"=w474, "Time to wait"=0.2, "Strin"=w468, "String in"=w467) -> ("error out"=w473:errorcluster, "Stopped"=w451:bool)  [unwired: 2 in]
                          n165 = call "Serial.vi"("error in (no error)"=w473, "write buffer"="EP=1\r\nVC=0\r\nMD[1]=0\r\n", "VISA resource name"=w458) -> ("error out"=w471:errorcluster)  [unwired: 7 in, 1 out]
                          n166 = call "RS232 DTR RTS.vi"("error in (no error)"=w471, "Func"=enum16{"Init", "VEnable", "PowerOnOff"}."PowerOnOff", "On/Off"=FALSE, "TesterCOM in"=w445) -> ("error out"=w470:errorcluster)  [unwired: 7 in]
                          n167 = call "Write panel message Kinetics (SubVI).vi"(4:"rpm"=w461, 5:"rpm"=FALSE ("rpm"), "PrintTime"=TRUE, "Stop"=w466, "error in (no error)"=w470, "Time to wait"=25.0, "Strin"=w468, "String in"=w467) -> ("error out"=w456:errorcluster, "Stopped"=w452:bool)  [unwired: 2 in]
                          n168 = call "RS232 DTR RTS.vi"("error in (no error)"=w456, "Func"=enum16{"Init", "VEnable", "PowerOnOff"}."PowerOnOff", "On/Off"=TRUE, "TesterCOM in"=w445) -> ("error out"=w455:errorcluster)  [unwired: 7 in]
                          n169 = call "RS232 DTR RTS.vi"("error in (no error)"=w455, "Func"=enum16{"Init", "VEnable", "PowerOnOff"}."VEnable", "On/Off"=TRUE, "TesterCOM in"=w445) -> ("error out"=w463:errorcluster)  [unwired: 7 in]
                          n170 = call "Write panel message Kinetics (SubVI).vi"(4:"rpm"=w461, 5:"rpm"=FALSE ("rpm"), "PrintTime"=TRUE, "Stop"=w466, "error in (no error)"=w463, "Time to wait"=3.0, "Strin"=w468, "String in"=w467) -> ("Stopped"=w453:bool)  [unwired: 2 in, 1 out]
                          n171 = Compound Arithmetic op=OR(w453, w452, w451) -> (w450:bool)
                          n172 = Compound Arithmetic op=OR(w453, w452, w451) -> (w460:bool)
                          n173 = Select(t=T5."Stop", s=w460, f=T5."FullSpeed1") -> (s? t:f=w486:T5)
                        }
                      }
                    }
                  }
                }
              }
            }
          }
        }
        frame "Venable Test" {
          n174 = control-ref of="Stop Button"() -> (w507:refnum<vi>)
          n175 = control-ref of="ATR"() -> (w508:refnum<vi>)
          n176 = control-ref of="Pannel User Message"() -> (w509:refnum<vi>)
          n177 = control-ref of="Motor Speed RPM Serial"() -> (w510:refnum<vi>)
          n178 = control-ref of="UUT"() -> (w511:refnum<vi>)
          n179 = Concatenate Strings(w503, " in process..." ("Strin")) -> (w504:string)
          n180 = while {
            shift-right: [w518] -> _
            shift-left: enum16{"Stop", "Direction", "Venable", "Start"}."Start" -> [w523]
            tunnel: w507 -> [w522]
            tunnel: w508 -> [w521]
            tunnel: w509 -> [w520]
            tunnel: w510 -> [w519]
            tunnel: w511 -> [w516]
            tunnel: w504 -> [w517]
            tunnel: w503 -> [w515]
            tunnel: w502 -> [w514]
            tunnel: [w512] -> w501
            stop <- w513 stop-if-true
            n181 = case shown="\"Start\"" w523 {
              tunnel: w522 -> [_ w553 w802 w850]
              tunnel: w521 -> [_ w549 w800 w843]
              tunnel: w520 -> [_ w552 w803 w856]
              tunnel: w519 -> [_ w551 w804 _]
              tunnel: w516 -> [w524 w545 w805 _]
              tunnel: [w526 FALSE FALSE FALSE] -> w513
              tunnel: [w525 w548 w801 w854] -> w518
              tunnel: w517 -> [_ w550 w799 w849]
              tunnel: w515 -> [_ _ _ w842]
              tunnel: w514 -> [_ _ _ w845]
              tunnel: [_ _ _ w837] -> w512
              frame "Stop", Default {
                n182 = disable-structure shown="Enabled" {
                  disable-tunnel: [w529 TRUE] -> w526
                  disable-tunnel: [w528 enum16{"Stop", "Direction", "Venable", "Start"}."Stop"] -> w525
                  disable-tunnel: w524 -> [w527 _]
                  frame Disabled {
                    n183 = flat-sequence {
                      tunnel: w527 -> [_]
                      tunnel: [TRUE] -> w529
                      tunnel: [enum16{"Stop", "Direction", "Venable", "Start"}."Stop"] -> w528
                      frame #0 {
                        (unwired) u16 0 ("Motor Speed RPM")
                        (unwired) TRUE ("Remote")
                        n184 = property on="VISA Kinetics" class="VISAName"() -> (error out=w533:errorcluster, "Value"=w534:refnum<visa-resource-name>)  [unwired: 2 in, 1 out]
                        n185 = call "Serial.vi"("error in (no error)"=w533, "Clear Log"=FALSE, "write buffer"="EP=1\r\nMD[1]=1\r\n", "VISA resource name"=w534) -> ("error out"=w530:errorcluster)  [unwired: 6 in, 1 out]
                        n186 = call "CANSendMessage.vi"("error in (no error)"=w530) -> ("error out"=w539:errorcluster)  [unwired: 10 in]
                        n187 = call "TesterOption (SubVI).vi"("2 Options"=FALSE, "error in (no error)"=w539, "On/Off"=FALSE, "Tester Option"=T6."Venable") -> ("error out"=w535:errorcluster)  [unwired: 6 in, 1 out]
                        n188 = call "Time Delay9"("error in (no error)"=w535) -> ()  [unwired: 10 in, 1 out]
                      }
                      frame #1 {
                      }
                    }
                  }
                  frame Enabled {
                  }
                }
              }
              frame "Direction" {
                n189 = property on="UUT" class="DigNum (strict)"() -> ("Value"=w544:u8)  [unwired: 2 in, 2 out]
                n190 = while {
                  shift-right: [w564] -> w547
                  shift-left: T5."MD[1]=0" -> [w565]
                  tunnel: w545 -> [w562]
                  tunnel: w553 -> [w561]
                  tunnel: w552 -> [w560]
                  tunnel: w551 -> [w559]
                  tunnel: w550 -> [w558]
                  tunnel: w549 -> [w557]
                  tunnel: w544 -> [w556]
                  stop <- w563 stop-if-true
                  n191 = case shown="\"MD[1]=0\"" w565 {
                    tunnel: [T5."Stop" w589 w626 w696 w724 w794] -> w564
                    tunnel: [TRUE FALSE FALSE FALSE FALSE FALSE] -> w563
                    tunnel: w562 -> [_ _ _ _ _ _]
                    tunnel: w561 -> [_ w576 w603 w666 w704 w762]
                    tunnel: w560 -> [_ _ w602 w675 w703 w772]
                    tunnel: w559 -> [_ _ w619 w664 w718 w768]
                    tunnel: w558 -> [_ _ w614 w683 w716 w780]
                    tunnel: w557 -> [_ w580 _ _ _ _]
                    tunnel: w556 -> [_ w568 w600 _ w698 _]
                    frame "Stop", Default {
                    }
                    frame "Result" {
                      n192 = property on="FullSpeed1 Current" class="DigNum (strict)"() -> ("Value"=w584:dbl)  [unwired: 2 in, 2 out]
                      n193 = property on="FullSpeed2 Current" class="DigNum (strict)"() -> ("Value"=w585:dbl)  [unwired: 2 in, 2 out]
                      n194 = property on="FullSpeed2 Speed" class="DigNum (strict)"() -> ("Value"=w587:dbl)  [unwired: 2 in, 2 out]
                      n195 = property on="FullSpeed1 Speed" class="DigNum (strict)"() -> ("Value"=w586:dbl)  [unwired: 2 in, 2 out]
                      n196 = Subtract(x=w585, y=w584) -> (x-y=w583:dbl)
                      n197 = Absolute Value(x=w583) -> (abs(x)=w572:dbl)
                      n198 = Greater Or Equal?(x=w572, y=u32 5) -> (x >= y?=w578:bool)
                      n199 = Equal?(x=w568, y=u8 95) -> (x = y?=w570:bool)
                      n200 = case shown="True" w570 {
                        tunnel: w587 -> [_ w598]
                        tunnel: w586 -> [_ w597]
                        tunnel: [TRUE w594] -> w579
                        frame False {
                        }
                        frame True {
                          n201 = Subtract(x=w598, y=w597) -> (x-y=w599:dbl)
                          n202 = Absolute Value(x=w599) -> (abs(x)=w596:dbl)
                          n203 = Greater Or Equal?(x=w596, y=500.0) -> (x >= y?=w594:bool)
                        }
                      }
                      n204 = call "Find_Number_LineMARVIN.vi"("Test Paragraph"="Motor Rotation Direction", "TableIn"=w580) -> ("Line number"=w577:i32)  [unwired: 3 in, 3 out]
                      n205 = And(x=w579, y=w578) -> (x .and. y?=w569:bool)
                      "VenableDirectionResult" <- w569
                      n206 = call "PassOrFail (SubVI).vi"("String Res"="", "index (row)"=w577, "Data in"=-3.0, "Pass?Fail"=w569, "Table in"=w580) -> ("error out"=w575:errorcluster)  [unwired: 6 in]
                      n207 = property class="Bool (strict)"(reference=w576, error in=w575) -> ("Value"=w592:bool)  [unwired: 2 out]
                      n208 = Select(t=T5."Stop", s=w592, f=T5."Stop") -> (s? t:f=w589:T5)
                    }
                    frame "FullSpeed2" {
                      (unwired) TRUE ("Remote")
                      n209 = Concatenate Strings(w614, "\nFull speed operation " ("string")) -> (w601:string)
                      n210 = call "CANSendMessage.vi"() -> ("error out"=w621:errorcluster)  [unwired: 11 in]
                      n211 = call "Write panel message Kinetics (SubVI).vi"(4:"rpm"=w619, 5:"rpm"=TRUE ("rpm"), "PrintTime"=FALSE, "Stop"=w603, "error in (no error)"=w621, "Time to wait"=0.2, "Strin"=w601, "String in"=w602) -> ("error out"=w606:errorcluster)  [unwired: 2 in, 1 out]
                      n212 = Equal?(x=w600, y=u8 95) -> (x = y?=w609:bool)
                      n213 = Select(t=u16 15100, s=w609, f=u16 12100 ("y")) -> ()  [unwired: 1 out]
                      n214 = flat-sequence {
                        tunnel: w606 -> [w631]
                        tunnel: [w631] -> w605
                        tunnel: [w630] -> w604
                        frame #0 {
                          n215 = call <vilib>:"High Resolution Relative Seconds.vi"() -> ("relative seconds"=w630:dbl)
                        }
                      }
                      n216 = Select(t=14500.0, s=w609, f=11500.0) -> (s? t:f=w608:dbl)
                      n217 = Select(t=47.0, s=w609, f=24.0) -> (s? t:f=w607:dbl)
                      n218 = while {
                        tunnel: w619 -> [w633]
                        tunnel: w605 -> [w657]
                        tunnel: [w640] -> w616
                        tunnel: w608 -> [w653]
                        tunnel: w607 -> [w652]
                        tunnel: w604 -> [w648]
                        tunnel: w603 -> [w638]
                        tunnel: w602 -> [w639]
                        tunnel: w601 -> [w636]
                        stop <- w650 stop-if-true
                        n219 = call <vilib>:"High Resolution Relative Seconds.vi"() -> ("relative seconds"=w649:dbl)
                        n220 = Subtract(x=w649, y=w648) -> (x-y=w647:dbl)
                        n221 = property class="DigNum (strict)"(reference=w633, error in=w657) -> ("Value"=w654:dbl)  [unwired: 2 out]
                        "FullSpeed2 Speed" <- w654
                        n222 = Greater Or Equal?(x=w647, y=120.0) -> (x >= y?=w645:bool)
                        n223 = Greater Or Equal?(x=w654, y=w653) -> (x >= y?=w644:bool)
                        n224 = property class="Bool (strict)"(reference=w638) -> ("Value"=w643:bool)  [unwired: 1 in, 2 out]
                        n225 = call "GetADCTester (SubVI).vi"("GetADCTester"=T7."Current", "TimeToGet"=5) -> ("error out"=w655:errorcluster, "ADCValOutput Single"=w651:dbl)  [unwired: 7 in, 1 out]
                        "FullSpeed2 Current" <- w651
                        n226 = Greater Or Equal?(x=w651, y=w652) -> (x >= y?=w641:bool)
                        n227 = And(x=w644, y=w641) -> (x .and. y?=w642:bool)
                        n228 = Compound Arithmetic op=OR(w643, w645, w642) -> (w650:bool)
                        n229 = call "Write panel message Kinetics (SubVI).vi"(4:"rpm"=w633, 5:"rpm"=TRUE ("rpm"), "PrintTime"=FALSE, "Stop"=w638, "error in (no error)"=w655, "Time to wait"=0.2, "Strin"=w636, "String in"=w639) -> ("error out"=w640:errorcluster)  [unwired: 2 in, 1 out]
                      }
                      n230 = property class="Bool (strict)"(reference=w603, error in=w616) -> ("Value"=w629:bool)  [unwired: 2 out]
                      n231 = Select(t=T5."Stop", s=w629, f=T5."Result") -> (s? t:f=w626:T5)
                    }
                    frame "MD[1]=1" {
                      (unwired) TRUE ("Remote")
                      (unwired) u16 0 ("Motor Speed RPM")
                      n232 = Concatenate Strings(w683, "\nSet Parameters MD[1]=1" ("Strin")) -> (w674:string)
                      n233 = call "TesterOption (SubVI).vi"("2 Options"=FALSE, "On/Off"=FALSE, "Tester Option"=T6."Venable") -> ("error out"=w688:errorcluster, "VISA Refnum out"=w679:refnum<visa-resource-name>)  [unwired: 7 in]
                      n234 = call "CANSendMessage.vi"("error in (no error)"=w688) -> ("error out"=w690:errorcluster)  [unwired: 10 in]
                      n235 = call "Write panel message Kinetics (SubVI).vi"(4:"rpm"=w664, 5:"rpm"=FALSE ("rpm"), "PrintTime"=TRUE, "Stop"=w666, "error in (no error)"=w690, "Time to wait"=20.0, "Strin"=w674, "String in"=w675) -> ("error out"=w663:errorcluster)  [unwired: 2 in, 1 out]
                      n236 = property on="VISA Kinetics" class="VISAName"(error in=w663) -> (error out=w689:errorcluster, "Value"=w692:refnum<visa-resource-name>)  [unwired: 1 in, 1 out]
                      n237 = call "Serial.vi"("error in (no error)"=w689, "Clear Log"=FALSE, "write buffer"="EP=1\r\nMD[1]=1\r\n", "VISA resource name"=w692) -> ("error out"=w678:errorcluster)  [unwired: 6 in, 1 out]
                      n238 = call "TesterOption (SubVI).vi"("2 Options"=FALSE, "error in (no error)"=w678, "On/Off"=FALSE, "Tester Option"=T6."Power", "VISA Refnum in"=w679) -> ("error out"=w676:errorcluster, "VISA Refnum out"=w667:refnum<visa-resource-name>)  [unwired: 5 in]
                      n239 = call "Write panel message Kinetics (SubVI).vi"(4:"rpm"=w664, 5:"rpm"=FALSE ("rpm"), "PrintTime"=TRUE, "Stop"=w666, "error in (no error)"=w676, "Time to wait"=25.0, "Strin"=w674, "String in"=w675) -> ("error out"=w668:errorcluster)  [unwired: 2 in, 1 out]
                      n240 = call "TesterOption (SubVI).vi"("2 Options"=FALSE, "error in (no error)"=w668, "On/Off"=TRUE, "Tester Option"=T6."Venable", "VISA Refnum in"=w667) -> ("error out"=w665:errorcluster)  [unwired: 5 in, 1 out]
                      n241 = call "Time Delay8"("error in (no error)"=w665) -> ("error out"=w661:errorcluster)  [unwired: 10 in]
                      n242 = property class="Bool (strict)"(reference=w666, error in=w661) -> ("Value"=w697:bool)  [unwired: 2 out]
                      n243 = Select(t=T5."Stop", s=w697, f=T5."FullSpeed2") -> (s? t:f=w696:T5)
                    }
                    frame "FullSpeed1" {
                      (unwired) TRUE ("Remote")
                      n244 = call "CANSendMessage.vi"() -> ("error out"=w719:errorcluster)  [unwired: 11 in]
                      n245 = Concatenate Strings(w716, "\nFull speed operation " ("string")) -> (w702:string)
                      n246 = call "Write panel message Kinetics (SubVI).vi"(4:"rpm"=w718, 5:"rpm"=TRUE ("rpm"), "PrintTime"=FALSE, "Stop"=w704, "error in (no error)"=w719, "Time to wait"=0.2, "Strin"=w702, "String in"=w703) -> ("error out"=w707:errorcluster)  [unwired: 2 in, 1 out]
                      n247 = Equal?(x=w698, y=u8 95) -> (x = y?=w714:bool)
                      n248 = flat-sequence {
                        tunnel: w707 -> [w729]
                        tunnel: [w729] -> w706
                        tunnel: [w728] -> w705
                        frame #0 {
                          n249 = call <vilib>:"High Resolution Relative Seconds.vi"() -> ("relative seconds"=w728:dbl)
                        }
                      }
                      n250 = Select(t=u16 15100, s=w714, f=u16 12100 ("y")) -> ()  [unwired: 1 out]
                      n251 = Select(t=13700.0, s=w714, f=11500.0) -> (s? t:f=w709:dbl)
                      n252 = Select(t=56.0, s=w714, f=33.0) -> (s? t:f=w708:dbl)
                      n253 = while {
                        tunnel: w718 -> [w731]
                        tunnel: w706 -> [w755]
                        tunnel: [w738] -> w717
                        tunnel: w709 -> [w750]
                        tunnel: w708 -> [w747]
                        tunnel: w705 -> [w745]
                        tunnel: w704 -> [w736]
                        tunnel: w703 -> [w737]
                        tunnel: w702 -> [w734]
                        stop <- w752 stop-if-true
                        n254 = property class="DigNum (strict)"(reference=w731, error in=w755) -> ("Value"=w751:dbl)  [unwired: 2 out]
                        "FullSpeed1 Speed" <- w751
                        n255 = call <vilib>:"High Resolution Relative Seconds.vi"() -> ("relative seconds"=w746:dbl)
                        n256 = Subtract(x=w746, y=w745) -> (x-y=w744:dbl)
                        n257 = Greater Or Equal?(x=w744, y=120.0) -> (x >= y?=w742:bool)
                        n258 = Greater Or Equal?(x=w751, y=w750) -> (x >= y?=w749:bool)
                        n259 = call "GetADCTester (SubVI).vi"("GetADCTester"=T7."Current", "TimeToGet"=5) -> ("error out"=w753:errorcluster, "ADCValOutput Single"=w748:dbl)  [unwired: 7 in, 1 out]
                        "FullSpeed1 Current" <- w748
                        n260 = Greater Or Equal?(x=w748, y=w747) -> (x >= y?=w739:bool)
                        n261 = And(x=w739, y=w749) -> (x .and. y?=w740:bool)
                        n262 = property class="Bool (strict)"(reference=w736) -> ("Value"=w741:bool)  [unwired: 1 in, 2 out]
                        n263 = call "Write panel message Kinetics (SubVI).vi"(4:"rpm"=w731, 5:"rpm"=TRUE ("rpm"), "PrintTime"=FALSE, "Stop"=w736, "error in (no error)"=w753, "Time to wait"=0.2, "Strin"=w734, "String in"=w737) -> ("error out"=w738:errorcluster)  [unwired: 2 in, 1 out]
                        n264 = Compound Arithmetic op=OR(w741, w740, w742) -> (w752:bool)
                      }
                      n265 = property class="Bool (strict)"(reference=w704, error in=w717) -> ("Value"=w727:bool)  [unwired: 2 out]
                      n266 = Select(t=T5."Stop", s=w727, f=T5."MD[1]=1") -> (s? t:f=w724:T5)
                    }
                    frame "MD[1]=0" {
                      (unwired) TRUE ("Remote")
                      (unwired) u16 0 ("Motor Speed RPM")
                      n267 = Concatenate Strings(w780, "\nSet Parameters MD[1]=0" ("Strin")) -> (w771:string)
                      n268 = call "TesterOption (SubVI).vi"("2 Options"=FALSE, "On/Off"=FALSE, "Tester Option"=T6."Venable") -> ("error out"=w786:errorcluster, "VISA Refnum out"=w776:refnum<visa-resource-name>)  [unwired: 7 in]
                      n269 = call "CANSendMessage.vi"("error in (no error)"=w786) -> ("error out"=w788:errorcluster)  [unwired: 10 in]
                      n270 = call "Write panel message Kinetics (SubVI).vi"(4:"rpm"=w768, 5:"rpm"=FALSE ("rpm"), "PrintTime"=FALSE, "Stop"=w762, "error in (no error)"=w788, "Time to wait"=0.2, "Strin"=w771, "String in"=w772) -> ("error out"=w783:errorcluster)  [unwired: 2 in, 1 out]
                      n271 = property on="VISA Kinetics" class="VISAName"(error in=w783) -> (error out=w787:errorcluster, "Value"=w790:refnum<visa-resource-name>)  [unwired: 1 in, 1 out]
                      n272 = call "Serial.vi"("error in (no error)"=w787, "Clear Log"=FALSE, "write buffer"="EP=1\r\nMD[1]=0\r\n", "VISA resource name"=w790) -> ("error out"=w775:errorcluster)  [unwired: 6 in, 1 out]
                      n273 = call "TesterOption (SubVI).vi"("2 Options"=FALSE, "error in (no error)"=w775, "On/Off"=FALSE, "Tester Option"=T6."Power", "VISA Refnum in"=w776) -> ("error out"=w773:errorcluster, "VISA Refnum out"=w763:refnum<visa-resource-name>)  [unwired: 5 in]
                      n274 = call "Write panel message Kinetics (SubVI).vi"(4:"rpm"=w768, 5:"rpm"=FALSE ("rpm"), "PrintTime"=TRUE, "Stop"=w762, "error in (no error)"=w773, "Time to wait"=25.0, "Strin"=w771, "String in"=w772) -> ("error out"=w764:errorcluster)  [unwired: 2 in, 1 out]
                      n275 = call "TesterOption (SubVI).vi"("2 Options"=FALSE, "error in (no error)"=w764, "On/Off"=TRUE, "Tester Option"=T6."Venable", "VISA Refnum in"=w763) -> ("error out"=w761:errorcluster)  [unwired: 5 in, 1 out]
                      n276 = call "Time Delay4"("error in (no error)"=w761) -> ("error out"=w757:errorcluster)  [unwired: 10 in]
                      n277 = property class="Bool (strict)"(reference=w762, error in=w757) -> ("Value"=w795:bool)  [unwired: 2 out]
                      n278 = Select(t=T5."Stop", s=w795, f=T5."FullSpeed1") -> (s? t:f=w794:T5)
                    }
                  }
                }
                n279 = flat-sequence {
                  tunnel: [enum16{"Stop", "Direction", "Venable", "Start"}."Stop"] -> w548
                  tunnel: w547 -> [_]
                  frame #0 {
                  }
                }
              }
              frame "Venable" {
                n280 = call "Find_Number_LineMARVIN.vi"("Test Paragraph"="Enable Test", "TableIn"=w800) -> ("Line number"=w806:i32)  [unwired: 3 in, 3 out]
                n281 = Increment(x=w806) -> (x+1=w796:i32)
                n282 = for {
                  tunnel: u16[] [5000, 0, 5000] -> [w831] mode=indexing
                  tunnel: bool[] [TRUE, FALSE, TRUE] -> [w829] mode=indexing
                  tunnel: w796 -> [w832]
                  tunnel: w805 -> [_]
                  tunnel: w804 -> [w822]
                  tunnel: w803 -> [w825]
                  tunnel: w802 -> [w824]
                  tunnel: w800 -> [w818]
                  tunnel: w799 -> [w816]
                  tunnel: [w815] -> w798 mode=indexing
                  i -> [w833]
                  (unwired) u16 5000 ("Motor Speed RPM")
                  (unwired) TRUE ("Remote")
                  w834 = 200.0 ("y")
                  n283 = call "CANSendMessage.vi"() -> ("error out"=w828:errorcluster)  [unwired: 11 in]
                  n284 = Add(x=w832, y=w833) -> (x+y=w819:i32)
                  n285 = call "TesterOption (SubVI).vi"("2 Options"=FALSE, "error in (no error)"=w828, "On/Off"=w829, "Tester Option"=T6."Venable") -> ("error out"=w827:errorcluster)  [unwired: 6 in, 1 out]
                  n286 = call "Write panel message Kinetics (SubVI).vi"(4:"rpm"=w822, 5:"rpm"=TRUE ("rpm"), "PrintTime"=TRUE, "Stop"=w824, "error in (no error)"=w827, "Time to wait"=15.0, "Strin"=w816, "String in"=w825) -> ("error out"=w826:errorcluster)  [unwired: 2 in, 1 out]
                  n287 = property class="DigNum (strict)"(reference=w822, error in=w826) -> ("Value"=w817:dbl)  [unwired: 2 out]
                  n288 = Add(x=w831, y=w834) -> (x+y=w836:dbl)
                  n289 = Subtract(x=w831, y=w834) -> (x-y=w835:dbl)
                  n290 = In Range and Coerce(upper limit=w836, x=w817, lower limit=w835) -> (In Range?=w815:bool)  [unwired: 1 out]
                  n291 = call "PassOrFail (SubVI).vi"("index (row)"=w819, "Data in"=w817, "Pass?Fail"=w815, "Table in"=w818) -> ()  [unwired: 7 in, 1 out]
                }
                n292 = property class="Bool (strict)"(reference=w802) -> ("Value"=w813:bool)  [unwired: 1 in, 2 out]
                n293 = And Array Elements(Boolean array=w798) -> (logical AND=→"VenableResult":bool)
                n294 = Select(t=enum16{"Stop", "Direction", "Venable", "Start"}."Stop", s=w813, f=enum16{"Stop", "Direction", "Venable", "Start"}."Direction") -> (s? t:f=w801:enum16{"Stop", "Direction", "Venable", "Start"})
              }
              frame "Start" {
                n295 = property class="Str"(reference=w856, "Value"=w849) -> (error out=w853:errorcluster)  [unwired: 1 in, 1 out]
                n296 = call "Find_Number_LineMARVIN.vi"("Test Paragraph"=w842, "error in"=w853, "TableIn"=w843) -> ("error out"=w844:errorcluster, "Line number"=w841:i32)  [unwired: 2 in, 2 out]
                n297 = call "Table_ScrollaBarMarvin.vi"("error in"=w844, "Line to focus"=w842, "reference in"=w843) -> ("error out"=w857:errorcluster)  [unwired: 2 out]
                n298 = call "Reset old test Values (SubVI) Kinetics.vi"("error in"=w857, "Atr in"=w843, "Test Paragraph"=w842) -> ("error out"=w838:errorcluster)  [unwired: 6 in, 2 out]
                n299 = Increment(x=w841) -> (x+1=w840:i32)
                n300 = while {
                  shift-right: [w869] -> _
                  shift-left: T4."VC=1000" -> [w872]
                  tunnel: w838 -> [w871]
                  tunnel: w845 -> [w870]
                  tunnel: w842 -> [w868]
                  shift-right: [w865] -> w848
                  shift-left: bool[] [FALSE, FALSE] -> [w866]
                  tunnel: w840 -> [w864]
                  tunnel: w843 -> [w863]
                  shift-right: [w861] -> _
                  shift-left: dbl[] [0.0, 0.0] -> [w862]
                  tunnel: [w859] -> w837
                  i -> [w867]
                  stop <- w860 stop-if-true
                  n301 = case shown="\"Exit\", Default" w872 {
                    tunnel: w871 -> [_ w890 _ w937 _]
                    tunnel: w870 -> [_ w889 w905 w940 _]
                    tunnel: [T4."Exit" T4."Wait" w902 T4."Wait" T4."ReadVC"] -> w869
                    tunnel: w868 -> [_ _ _ _ w947]
                    tunnel: [TRUE FALSE FALSE FALSE w942] -> w860
                    tunnel: w867 -> [_ _ w903 _ _]
                    tunnel: w866 -> [w874 w887 w901 w938 w944]
                    tunnel: [w874 w887 w900 w938 w944] -> w865
                    tunnel: w864 -> [w875 _ _ _ _]
                    tunnel: w863 -> [w876 _ _ _ _]
                    tunnel: w862 -> [w873 w885 w898 w933 w943]
                    tunnel: [w873 w885 w897 w933 w943] -> w861
                    tunnel: [_ _ _ _ w942] -> w859
                    frame "Exit", Default {
                      n302 = for {
                        tunnel: w876 -> [w884]
                        tunnel: w875 -> [w883]
                        tunnel: w874 -> [w882] mode=indexing
                        tunnel: w873 -> [w879] mode=indexing
                        i -> [w880]
                        n303 = Add(x=w880, y=w883) -> (x+y=w881:i32)
                        n304 = call "PassOrFail (SubVI).vi"("index (row)"=w881, "Data in"=w879, "Pass?Fail"=w882, "Table in"=w884) -> ()  [unwired: 7 in, 1 out]
                      }
                    }
                    frame "VC=0" {
                      n305 = disable-structure shown="Enabled" {
                        disable-tunnel: w890 -> [w893 _]
                        disable-tunnel: w889 -> [w891 _]
                        frame Disabled {
                          n306 = call "Serial.vi"("error in (no error)"=w893, "write buffer"="EP=1\r\nVC=0\r\n", "VISA resource name"=w891) -> ()  [unwired: 7 in, 2 out]
                        }
                        frame Enabled {
                          n307 = local read "TesterCOM"() -> (w895:refnum<visa-resource-name>)
                          n308 = call "RS232 DTR RTS.vi"("Func"=enum16{"Init", "VEnable", "PowerOnOff"}."VEnable", "On/Off"=FALSE, "TesterCOM in"=w895) -> ()  [unwired: 8 in, 1 out]
                        }
                      }
                    }
                    frame "ReadVC" {
                      n309 = call "Serial.vi"("write buffer"="VC\r\n", "VISA resource name"=w905) -> ("read buffer"=w904:string)  [unwired: 8 in, 1 out]
                      n310 = case shown="2" w903 {
                        tunnel: w904 -> [w917 w927]
                        tunnel: [T4."VC=0" T4."Exit"] -> w902
                        tunnel: w901 -> [w913 w926]
                        tunnel: [w911 w923] -> w900
                        tunnel: w898 -> [w910 w922]
                        tunnel: [w907 w919] -> w897
                        frame 2 {
                          n311 = Decimal String To Number(string=w917) -> (number=w908:i32)  [unwired: 2 in, 1 out]
                          n312 = In Range and Coerce(upper limit=1100, x=w908, lower limit=900) -> (In Range?=w912:bool)  [unwired: 1 out]
                          n313 = Replace Array Subset(array=w910, new element=w908, index=0) -> (w907:dbl[])
                          n314 = Replace Array Subset(array=w913, new element=w912, index=0) -> (w911:bool[])
                        }
                        frame 5, Default {
                          n315 = Decimal String To Number(string=w927) -> (number=w920:i32)  [unwired: 2 in, 1 out]
                          n316 = In Range and Coerce(upper limit=100, x=w920, lower limit=0) -> (In Range?=w924:bool)  [unwired: 1 out]
                          n317 = Replace Array Subset(array=w922, new element=w920, index=1) -> (w919:dbl[])
                          n318 = Replace Array Subset(array=w926, new element=w924, index=1) -> (w923:bool[])
                        }
                      }
                    }
                    frame "VC=1000" {
                      n319 = local read "TesterCOM"() -> (w932:refnum<visa-resource-name>)
                      n320 = call "RS232 DTR RTS.vi"("error in (no error)"=w937, "Func"=enum16{"Init", "VEnable", "PowerOnOff"}."VEnable", "On/Off"=TRUE, "TesterCOM in"=w932) -> ("error out"=w936:errorcluster)  [unwired: 7 in]
                      n321 = call "Serial.vi"("error in (no error)"=w936, "write buffer"="EP=1\r\nVC=1000\r\n", "VISA resource name"=w940) -> ()  [unwired: 7 in, 2 out]
                    }
                    frame "Wait" {
                      n322 = control-ref of="Motor Speed RPM Serial"() -> (w952:refnum<vi>)
                      n323 = control-ref of="Pannel User Message"() -> (w951:refnum<vi>)
                      n324 = control-ref of="Stop Button"() -> (w946:refnum<vi>)
                      n325 = call "Write panel message Kinetics (SubVI).vi"(4:"rpm"=w952, 5:"rpm"=TRUE ("rpm"), "PrintTime"=TRUE, "Stop"=w946, "Time to wait"=20.0, "Strin"=w947, "String in"=w951) -> ("Stopped"=w942:bool)  [unwired: 3 in, 1 out]
                    }
                  }
                }
                n326 = And Array Elements(Boolean array=w848) -> ()  [unwired: 1 out]
                n327 = property class="Bool (strict)"(reference=w850) -> ("Value"=w858:bool)  [unwired: 1 in, 2 out]
                n328 = Select(t=enum16{"Stop", "Direction", "Venable", "Start"}."Stop", s=w858, f=enum16{"Stop", "Direction", "Venable", "Start"}."Stop") -> (s? t:f=w854:enum16{"Stop", "Direction", "Venable", "Start"})
              }
            }
          }
        }
        frame "Motor Thermistor Test" {
          n329 = Concatenate Strings(w964, " in process..." ("Strin")) -> (w965:string)
          n330 = control-ref of="ATR"() -> (w967:refnum<vi>)
          n331 = control-ref of="Pannel User Message"() -> (w968:refnum<vi>)
          n332 = property class="Str"(reference=w968, "Value"=w965) -> (error out=w961:errorcluster)  [unwired: 1 in, 1 out]
          n333 = call "Find_Number_LineMARVIN.vi"("Test Paragraph"=w964, "error in"=w961, "TableIn"=w967) -> ("error out"=w958:errorcluster, "Line number"=w957:i32)  [unwired: 2 in, 2 out]
          n334 = call "Table_ScrollaBarMarvin.vi"("error in"=w958, "Line to focus"=w964, "reference in"=w967) -> ("error out"=w962:errorcluster)  [unwired: 2 out]
          n335 = call "Reset old test Values (SubVI) Kinetics.vi"("error in"=w962, "Atr in"=w967, "Test Paragraph"=w964) -> ("error out"=w954:errorcluster)  [unwired: 6 in, 2 out]
          n336 = Increment(x=w957) -> (x+1=w956:i32)
          n337 = while {
            shift-right: [w979] -> _
            shift-left: T4."VC=1000" -> [w982]
            tunnel: w954 -> [w981]
            tunnel: w963 -> [w980]
            tunnel: w964 -> [w978]
            shift-right: [w974] -> _
            shift-left: bool[] [FALSE, FALSE] -> [w975]
            tunnel: w956 -> [w973]
            tunnel: w967 -> [w972]
            shift-right: [w970] -> _
            shift-left: dbl[] [0.0, 0.0] -> [w971]
            tunnel: [w969] -> w953
            i -> [w976]
            stop <- w977 stop-if-true
            n338 = case shown="\"Exit\", Default" w982 {
              tunnel: w981 -> [_ w1007 _ w1068 _]
              tunnel: w980 -> [w986 w1006 w1026 w1071 _]
              tunnel: [T4."Exit" T4."Wait" w1023 T4."Wait" T4."ReadVC"] -> w979
              tunnel: w978 -> [_ _ _ _ w1078]
              tunnel: [TRUE FALSE FALSE FALSE w1073] -> w977
              tunnel: w976 -> [_ w1001 w1024 _ _]
              tunnel: w975 -> [w990 w1004 w1022 w1069 w1075]
              tunnel: [w990 w1004 w1021 w1069 w1075] -> w974
              tunnel: w973 -> [w991 _ _ _ _]
              tunnel: w972 -> [w992 _ _ _ _]
              tunnel: w971 -> [w989 w1002 w1019 w1064 w1074]
              tunnel: [w989 w1002 w1018 w1064 w1074] -> w970
              tunnel: [_ _ _ _ w1073] -> w969
              frame "Exit", Default {
                n339 = for {
                  tunnel: w992 -> [w1000]
                  tunnel: w991 -> [w999]
                  tunnel: w990 -> [w998] mode=indexing
                  tunnel: w989 -> [w995] mode=indexing
                  i -> [w996]
                  n340 = Add(x=w996, y=w999) -> (x+y=w997:i32)
                  n341 = call "PassOrFail (SubVI).vi"("index (row)"=w997, "Data in"=w995, "Pass?Fail"=w998, "Table in"=w1000) -> ()  [unwired: 7 in, 1 out]
                }
                n342 = local read "TesterCOM"() -> (w985:refnum<visa-resource-name>)
                n343 = call "Serial.vi"("write buffer"="EP=1\r\nVC=0\r\n", "VISA resource name"=w986) -> ("error out"=w983:errorcluster)  [unwired: 8 in, 1 out]
                n344 = call "RS232 DTR RTS.vi"("error in (no error)"=w983, "Func"=enum16{"Init", "VEnable", "PowerOnOff"}."VEnable", "On/Off"=FALSE, "TesterCOM in"=w985) -> ()  [unwired: 7 in, 1 out]
              }
              frame "VC=0" {
                n345 = disable-structure shown="Enabled" {
                  disable-tunnel: w1007 -> [_ _]
                  disable-tunnel: w1006 -> [_ _]
                  disable-tunnel: w1001 -> [w1008 w1014]
                  frame Enabled {
                    n346 = case shown="6, Default" w1008 {
                      tunnel: [TRUE ("On/Off") FALSE ("On/Off")] -> w1009
                      frame 6, Default {
                      }
                      frame 3 {
                      }
                    }
                    n347 = local read "TesterCOM"() -> (w1011:refnum<visa-resource-name>)
                    n348 = call "RS232 DTR RTS.vi"("Func"=enum16{"Init", "VEnable", "PowerOnOff"}."VEnable", "On/Off"=w1009, "TesterCOM in"=w1011) -> ()  [unwired: 8 in, 1 out]
                  }
                  frame Disabled {
                    n349 = case shown="3" w1014 {
                      tunnel: ["Connect wires of the thermistor" ("message") "Disconnect wires of the thermistor" ("message")] -> w1015
                      frame 6, Default {
                      }
                      frame 3 {
                      }
                    }
                    n350 = One Button Dialog(message=w1015) -> ()  [unwired: 1 in, 1 out]
                  }
                }
              }
              frame "ReadVC" {
                n351 = call "Serial.vi"("write buffer"="VC\r\n", "VISA resource name"=w1026) -> ("read buffer"=w1025:string)  [unwired: 8 in, 1 out]
                n352 = case shown="8" w1024 {
                  tunnel: w1025 -> [w1037 w1046 w1058]
                  tunnel: [w1031 T4."VC=0" T4."Exit"] -> w1023
                  tunnel: w1022 -> [w1028 w1045 w1057]
                  tunnel: [w1028 w1042 w1054] -> w1021
                  tunnel: w1019 -> [w1029 w1041 w1053]
                  tunnel: [w1029 w1038 w1050] -> w1018
                  frame 2 {
                    n353 = Decimal String To Number(string=w1037) -> (number=w1034:i32)  [unwired: 2 in, 1 out]
                    n354 = In Range and Coerce(upper limit=1100, x=w1034, lower limit=900) -> (In Range?=w1033:bool)  [unwired: 1 out]
                    n355 = Select(t=T4."VC=0", s=w1033, f=T4."Exit") -> (s? t:f=w1031:T4)
                  }
                  frame 5, Default {
                    n356 = Decimal String To Number(string=w1046) -> (number=w1039:i32)  [unwired: 2 in, 1 out]
                    n357 = In Range and Coerce(upper limit=100, x=w1039, lower limit=0) -> (In Range?=w1043:bool)  [unwired: 1 out]
                    n358 = Replace Array Subset(array=w1041, new element=w1039, index=0) -> (w1038:dbl[])
                    n359 = Replace Array Subset(array=w1045, new element=w1043, index=0) -> (w1042:bool[])
                  }
                  frame 8 {
                    n360 = Decimal String To Number(string=w1058) -> (number=w1051:i32)  [unwired: 2 in, 1 out]
                    n361 = In Range and Coerce(upper limit=1100, x=w1051, lower limit=900) -> (In Range?=w1055:bool)  [unwired: 1 out]
                    n362 = Replace Array Subset(array=w1053, new element=w1051, index=1) -> (w1050:dbl[])
                    n363 = Replace Array Subset(array=w1057, new element=w1055, index=1) -> (w1054:bool[])
                  }
                }
              }
              frame "VC=1000" {
                n364 = local read "TesterCOM"() -> (w1063:refnum<visa-resource-name>)
                n365 = call "RS232 DTR RTS.vi"("error in (no error)"=w1068, "Func"=enum16{"Init", "VEnable", "PowerOnOff"}."VEnable", "On/Off"=TRUE, "TesterCOM in"=w1063) -> ("error out"=w1067:errorcluster)  [unwired: 7 in]
                n366 = call "Serial.vi"("error in (no error)"=w1067, "write buffer"="EP=1\r\nVC=1000\r\n", "VISA resource name"=w1071) -> ()  [unwired: 7 in, 2 out]
              }
              frame "Wait" {
                n367 = control-ref of="Motor Speed RPM Serial"() -> (w1083:refnum<vi>)
                n368 = control-ref of="Pannel User Message"() -> (w1082:refnum<vi>)
                n369 = control-ref of="Stop Button"() -> (w1077:refnum<vi>)
                n370 = call "Write panel message Kinetics (SubVI).vi"(4:"rpm"=w1083, 5:"rpm"=TRUE ("rpm"), "PrintTime"=TRUE, "Stop"=w1077, "Time to wait"=20.0, "Strin"=w1078, "String in"=w1082) -> ("Stopped"=w1073:bool)  [unwired: 3 in, 1 out]
              }
            }
          }
        }
        frame "Motor Run Test" {
          n371 = control-ref of="Pannel User Message"() -> (w1103:refnum<vi>)
          n372 = Concatenate Strings(w1087, " in process..." ("Strin")) -> (w1092:string)
          n373 = property class="Str"(reference=w1103, error in=w1100, "Value"=w1092) -> (error out=w1102:errorcluster)  [unwired: 1 out]
          n374 = call "Table_ScrollaBarMarvin.vi"("error in"=w1102, "Line to focus"=w1087, "reference in"=w1095) -> ()  [unwired: 3 out]
          n375 = call "Reset old test Values (SubVI) Kinetics.vi"("Atr in"=w1095, "Test Paragraph"=w1087) -> ("error out"=w1101:errorcluster)  [unwired: 7 in, 2 out]
          n376 = call "Find_Number_LineMARVIN.vi"("Test Paragraph"=w1087, "error in"=w1101, "TableIn"=w1095) -> ("error out"=w1098:errorcluster, "Line number"=w1094:i32)  [unwired: 2 in, 2 out]
          n377 = Increment(x=w1094) -> (x+1=w1093:i32)
          n378 = while {
            tunnel: w1098 -> [w1106]
            tunnel: w1088 -> [w1113]
            shift-right: [w1111] -> _
            shift-left: T8."Init" -> [w1112]
            tunnel: w1095 -> [w1110]
            tunnel: w1093 -> [w1109]
            tunnel: w1092 -> [w1107]
            tunnel: [w1106] -> w1089
            tunnel: [w1104] -> w1086
            i -> [w1108]
            stop <- w1105 stop-if-true
            n379 = case shown="\"Exit\", Default" w1112 {
              tunnel: w1106 -> [_ w1119 w1140 w1177 w1195]
              tunnel: w1113 -> [_ _ _ w1178 _]
              tunnel: [T8."Exit" T8."ReadTemp" w1137 T8."ReadCurrent" T8."ReadTemp"] -> w1111
              tunnel: w1110 -> [_ _ w1151 w1172 _]
              tunnel: w1109 -> [_ _ w1153 w1174 _]
              tunnel: w1108 -> [_ _ w1154 w1175 _]
              tunnel: w1107 -> [_ w1120 w1139 _ _]
              tunnel: [TRUE ("Stopped") w1117 w1133 _ _] -> w1105
              tunnel: [_ w1117 _ _ _] -> w1104
              frame "Exit", Default {
              }
              frame "Wait" {
                n380 = control-ref of="Motor Speed RPM Serial"() -> (w1125:refnum<vi>)
                n381 = control-ref of="Pannel User Message"() -> (w1124:refnum<vi>)
                n382 = control-ref of="Stop Button"() -> (w1123:refnum<vi>)
                n383 = call "Write panel message Kinetics (SubVI).vi"(4:"rpm"=w1125, 5:"rpm"=TRUE ("rpm"), "PrintTime"=TRUE, "Stop"=w1123, "error in (no error)"=w1119, "Time to wait"=1140.0, "Strin"=w1120, "String in"=w1124) -> ("Stopped"=w1117:bool)  [unwired: 2 in, 1 out]
              }
              frame "ReadCurrent" {
                w1149 = 3.0 ("x")
                n384 = control-ref of="Motor Speed RPM Serial"() -> (w1146:refnum<vi>)
                n385 = control-ref of="Pannel User Message"() -> (w1145:refnum<vi>)
                n386 = control-ref of="Stop Button"() -> (w1144:refnum<vi>)
                n387 = call "Write panel message Kinetics (SubVI).vi"(4:"rpm"=w1146, 5:"rpm"=TRUE ("rpm"), "PrintTime"=TRUE, "Stop"=w1144, "error in (no error)"=w1140, "Time to wait"=59.0, "Strin"=w1139, "String in"=w1145) -> ("error out"=w1136:errorcluster, "Stopped"=w1138:bool)  [unwired: 2 in]
                n388 = property on="UUT" class="Str"() -> ("Value"=w1135:string)  [unwired: 2 in, 2 out]
                n389 = case shown="\"True\", Default" w1135 {
                  tunnel: [w1155 w1157] -> w1134
                  tunnel: w1136 -> [_ _]
                  frame "Condenser India", "Condenser Merkava" {
                    n390 = call "Current prob"() -> ("Current"=w1155:dbl)  [unwired: 17 in, 2 out]
                  }
                  frame "True", Default {
                    n391 = local read "CurrentOut"() -> (w1156:dbl)
                    n392 = To Double Precision Float(number=w1156) -> (double precision float=w1157:dbl)
                  }
                }
                n393 = case shown="2, Default" w1154 {
                  tunnel: w1153 -> [w1160 w1163]
                  tunnel: [w1159 w1164] -> w1152
                  tunnel: [T8."Wait" T8."Exit"] -> w1137
                  frame 2, Default {
                    n394 = Increment(x=w1160) -> (x+1=w1159:i32)
                  }
                  frame 5 {
                    n395 = Add(x=w1163, y=3) -> (x+y=w1164:i32)
                  }
                }
                n396 = call "ValFromATR(SubVI).vi"("Row"=w1152, "Table in"=w1151) -> ("Val"=w1150:dbl)  [unwired: 8 in, 1 out]
                n397 = Add(x=w1149, y=w1150) -> (x+y=w1148:dbl)
                n398 = Subtract(x=w1150, y=w1149) -> (x-y=w1147:dbl)
                n399 = local read "TesterCOM"() -> (w1127:refnum<visa-resource-name>)
                n400 = In Range and Coerce(upper limit=w1148, x=w1134, lower limit=w1147) -> (In Range?=w1130:bool)  [unwired: 1 out]
                n401 = Not(x=w1130) -> (.not. x?=w1132:bool)
                n402 = Compound Arithmetic op=OR(w1138, w1132) -> (w1133:bool)
                n403 = Not(x=w1130) -> (.not. x?=w1131:bool)
                n404 = call "PassOrFail (SubVI).vi"("index (row)"=w1152, "Data in"=w1134, "Pass?Fail"=w1130, "Table in"=w1151) -> ("error out"=w1128:errorcluster)  [unwired: 7 in]
                n405 = call "RS232 DTR RTS.vi"("error in (no error)"=w1128, "Func"=enum16{"Init", "VEnable", "PowerOnOff"}."PowerOnOff", "On/Off"=w1130, "TesterCOM in"=w1127) -> ("error out"=w1129:errorcluster)  [unwired: 7 in]
                n406 = call "Display Message to User7"("error in (no error)"=w1129, "Enable"=w1131) -> ()  [unwired: 8 in, 2 out]
              }
              frame "ReadTemp" {
                w1170 = 15.0 ("x")
                n407 = case shown="4" w1175 {
                  tunnel: w1174 -> [w1180 w1182]
                  tunnel: [w1180 w1183] -> w1173
                  frame 1, Default {
                  }
                  frame 4 {
                    n408 = Add(x=w1182, y=2) -> (x+y=w1183:i32)
                  }
                }
                n409 = call "Serial.vi"("error in (no error)"=w1177, "write buffer"="TA[1]\r\n", "VISA resource name"=w1178) -> ("read buffer"=w1176:string)  [unwired: 7 in, 1 out]
                n410 = call "ValFromATR(SubVI).vi"("Row"=w1173, "Table in"=w1172) -> ("Val"=w1171:dbl)  [unwired: 8 in, 1 out]
                n411 = Fract/Exp String To Number(string=w1176) -> (number=w1166:dbl)  [unwired: 3 in, 1 out]
                n412 = Add(x=w1170, y=w1171) -> (x+y=w1169:dbl)
                n413 = Subtract(x=w1171, y=w1170) -> (x-y=w1168:dbl)
                n414 = In Range and Coerce(upper limit=w1169, x=w1166, lower limit=w1168) -> (In Range?=w1167:bool)  [unwired: 1 out]
                n415 = call "PassOrFail (SubVI).vi"("index (row)"=w1173, "Data in"=w1166, "Pass?Fail"=w1167, "Table in"=w1172) -> ()  [unwired: 7 in, 1 out]
              }
              frame "Init" {
                n416 = local read "TesterCOM"() -> (w1192:refnum<visa-resource-name>)
                n417 = call "RS232 DTR RTS.vi"("error in (no error)"=w1195, "Func"=enum16{"Init", "VEnable", "PowerOnOff"}."PowerOnOff", "On/Off"=FALSE, "TesterCOM in"=w1192) -> ("error out"=w1194:errorcluster)  [unwired: 7 in]
                n418 = call "Time Delay15"("error in (no error)"=w1194) -> ("error out"=w1187:errorcluster)  [unwired: 10 in]
                n419 = local read "TesterCOM"() -> (w1186:refnum<visa-resource-name>)
                n420 = call "RS232 DTR RTS.vi"("error in (no error)"=w1187, "Func"=enum16{"Init", "VEnable", "PowerOnOff"}."VEnable", "On/Off"=TRUE, "TesterCOM in"=w1186) -> ("error out"=w1185:errorcluster)  [unwired: 7 in]
                n421 = local read "TesterCOM"() -> (w1190:refnum<visa-resource-name>)
                n422 = call "RS232 DTR RTS.vi"("error in (no error)"=w1185, "Func"=enum16{"Init", "VEnable", "PowerOnOff"}."PowerOnOff", "On/Off"=TRUE, "TesterCOM in"=w1190) -> ("error out"=w1184:errorcluster)  [unwired: 7 in]
                n423 = call "Time Delay2"("error in (no error)"=w1184) -> ()  [unwired: 10 in, 1 out]
              }
            }
          }
          n424 = call "Serial.vi"("error in (no error)"=w1089, "write buffer"="EP=1\r\nVC=0\r\n", "VISA resource name"=w1088) -> ("error out"=w1090:errorcluster)  [unwired: 7 in, 1 out]
          n425 = local read "TesterCOM"() -> (w1085:refnum<visa-resource-name>)
          n426 = call "RS232 DTR RTS.vi"("error in (no error)"=w1090, "Func"=enum16{"Init", "VEnable", "PowerOnOff"}."VEnable", "On/Off"=FALSE, "TesterCOM in"=w1085) -> ()  [unwired: 7 in, 1 out]
        }
        frame "Set Production Parameters" {
          n427 = control-ref of="Pannel User Message"() -> (w1218:refnum<vi>)
          n428 = Concatenate Strings(w1211, " in process..." ("Strin")) -> (w1215:string)
          n429 = property class="Str"(reference=w1218, error in=w1213, "Value"=w1215) -> (error out=w1217:errorcluster)  [unwired: 1 out]
          n430 = call "Table_ScrollaBarMarvin.vi"("error in"=w1217, "Line to focus"=w1211, "reference in"=w1209) -> ("error out"=w1212:errorcluster)  [unwired: 2 out]
          n431 = call "Reset old test Values (SubVI) Kinetics.vi"("error in"=w1212, "Atr in"=w1209, "Test Paragraph"=w1211) -> ("error out"=w1216:errorcluster)  [unwired: 6 in, 2 out]
          n432 = call "Find_Number_LineMARVIN.vi"("Test Paragraph"=w1211, "error in"=w1216, "TableIn"=w1209) -> ("error out"=w1202:errorcluster, "Line number"=w1207:i32)  [unwired: 2 in, 2 out]
          n433 = local read "TesterCOM"() -> (w1200:refnum<visa-resource-name>)
          n434 = call "RS232 DTR RTS.vi"("error in (no error)"=w1202, "Func"=enum16{"Init", "VEnable", "PowerOnOff"}."PowerOnOff", "On/Off"=TRUE, "TesterCOM in"=w1200) -> ("error out"=w1204:errorcluster)  [unwired: 7 in]
          n435 = call "Time Delay16"("error in (no error)"=w1204) -> ("error out"=w1201:errorcluster)  [unwired: 10 in]
          n436 = Increment(x=w1207) -> (x+1=w1206:i32)
          n437 = for {
            tunnel: w1210 -> [w1227]
            tunnel: w1209 -> [w1226]
            tunnel: w1201 -> [w1225]
            tunnel: string[] ["SN\r\n", "PN\r\n"] -> [w1223] mode=indexing
            tunnel: w1206 -> [w1220]
            i -> [w1221]
            n438 = call "Serial.vi"("error in (no error)"=w1225, "write buffer"=w1223, "VISA resource name"=w1227) -> ("error out"=w1224:errorcluster, "read buffer"=w1222:string)  [unwired: 7 in]
            n439 = Add(x=w1220, y=w1221) -> (x+y=w1219:i32)
            n440 = case shown="0, Default" w1221 {
              tunnel: w1226 -> [w1236 w1243]
              tunnel: w1224 -> [w1235 w1242]
              tunnel: w1222 -> [w1228 w1238]
              tunnel: w1219 -> [w1229 w1237]
              frame 0, Default {
                n441 = property on="Next SN" class="DigNum (strict)"() -> ("Value"=w1233:i32)  [unwired: 2 in, 2 out]
                n442 = Decrement(x=w1233) -> (x-1=w1234:i32)
                n443 = Number To Decimal String(number=w1234) -> (decimal integer string=w1232:string)  [unwired: 1 in]
                n444 = Equal?(x=w1228, y=w1232) -> (x = y?=w1231:bool)
                n445 = call "PassOrFail (SubVI).vi"("String Res"=w1228, "index (row)"=w1229, "error in (no error)"=w1235, "Data in"=-3.0, "Pass?Fail"=w1231, "Table in"=w1236) -> ()  [unwired: 5 in, 1 out]
              }
              frame 1 {
                n446 = property on="PN" class="Str"() -> ("Value"=w1241:string)  [unwired: 2 in, 2 out]
                n447 = Equal?(x=w1241, y=w1238) -> (x = y?=w1240:bool)
                n448 = call "PassOrFail (SubVI).vi"("String Res"=w1238, "index (row)"=w1237, "error in (no error)"=w1242, "Data in"=-3.0, "Pass?Fail"=w1240, "Table in"=w1243) -> ()  [unwired: 5 in, 1 out]
              }
            }
          }
        }
      }
      "TestinExecution" <- w63
    }
    n449 = flat-sequence {
      tunnel: w47 -> [_]
      frame #0 {
        w57 = T9."Enabled" ("Disabled")
        w58 = FALSE ("Start")
        n450 = property on="Start" class="Bool (strict)"("Value"=w58, "DisabledEnum"=w57) -> ()  [unwired: 2 in, 2 out]
        n451 = local read "TesterCOM"() -> (w55:refnum<visa-resource-name>)
        n452 = property on="Report" class="Bool (strict)"("Value"=w58, "DisabledEnum"=w57) -> ()  [unwired: 2 in, 2 out]
        n453 = call "RS232 DTR RTS.vi"("Func"=enum16{"Init", "VEnable", "PowerOnOff"}."PowerOnOff", "On/Off"=FALSE, "TesterCOM in"=w55) -> ()  [unwired: 8 in, 1 out]
      }
    }
  }
  n454 = while {
    shift-right: [w1248] -> _
    shift-left: T2."Initialize" -> [w1263]
    shift-right: [w1260] -> _
    shift-left: _ -> [w1259]
    shift-right: [w1257] -> _
    shift-left: w25 -> [w1258]
    tunnel: "ATR" -> [_]
    tunnel: w20 -> [w1256]
    tunnel: w19 -> [w1255]
    shift-right: [w1253] -> _
    shift-left: w3 -> [w1254]
    tunnel: w10 -> [w1252]
    tunnel: w4 -> [w1251]
    tunnel: w18 -> [_]
    tunnel: w1 -> [w1262]
    tunnel: [w1261] -> _
    tunnel: w11 -> [_]
    tunnel: w8 -> [w1249]
    shift-right: [w1246] -> _
    shift-left: w3 -> [w1247]
    shift-right: [w1244] -> _
    shift-left: w3 -> [w1245]
    stop <- w1250 stop-if-true
    n455 = case shown="\"Erase ATR Table\", Default" w1263 {
      tunnel: [T2."MainProgram" w1450 w1499 T2."Erase ATR Table"] -> w1248
      tunnel: [FALSE w1440 FALSE FALSE] -> w1250
      tunnel: [w1301 w1444 w1493 w1929] -> w1261
      tunnel: w1262 -> [_ w1418 w1497 _]
      tunnel: [w1276 refnum<visa-resource-name> refnum ("VISA resource name") w1494 w1926] -> w1260
      tunnel: w1259 -> [_ w1460 w1495 _]
      tunnel: w1258 -> [w1315 w1456 w1492 w1945]
      tunnel: [w1315 w1434 w1491 w1945] -> w1257
      tunnel: w1256 -> [_ _ w1490 _]
      tunnel: w1255 -> [_ _ w1489 _]
      tunnel: w1254 -> [w1313 w1454 w1488 w1943]
      tunnel: [w1313 w1454 w1487 w1943] -> w1253
      tunnel: w1252 -> [w1312 _ w1486 _]
      tunnel: w1251 -> [_ _ w1485 _]
      tunnel: w1249 -> [_ _ w1484 _]
      tunnel: w1247 -> [_ _ w1483 _]
      tunnel: [w1309 w1433 w1482 w1939] -> w1246
      tunnel: w1245 -> [_ _ w1481 _]
      tunnel: [w1309 w1433 w1480 w1939] -> w1244
      frame "Erase ATR Table", Default {
        w1303 = refnum<visa-resource-name> "COMx" ("VISA Kinetics")
        w1309 = 0
        w1311 = T9."Enabled" ("Disabled")
        w1317 = FALSE ("Visible")
        n456 = property on="Serial Com" class="Bool"(error in=errorcluster {"status"=FALSE, "code"=0, "source"=""} ("error out"), "Visible"=FALSE) -> (error out=w1314:errorcluster)  [unwired: 1 in, 1 out]
        n457 = property on="VISA Kinetics" class="VISAName"(error in=w1314, "Visible"=w1317, "Value"=w1303) -> (error out=w1319:errorcluster)  [unwired: 1 in, 1 out]
        n458 = property on="Serial Status" class="Bool (strict)"(error in=w1319, "Value"=w1317) -> (error out=w1307:errorcluster)  [unwired: 1 in, 1 out]
        n459 = property on="Pannel User Message" class="Str"(error in=w1307, "Value"="Select a UUT from list bellow:") -> (error out=w1273:errorcluster)  [unwired: 1 in, 1 out]
        n460 = while {
          tunnel: [w1340] -> w1275
          tunnel: w1273 -> [w1339]
          tunnel: [w1338] -> w1272
          stop <- w1343 stop-if-true
          n461 = call "UUT Select"("error in (no error)"=w1339) -> ("India"=w1337:bool, "Merkava"=w1336:bool, "OK"=w1335:bool, "error out"=w1338:errorcluster)  [unwired: 15 in]
          n462 = Exclusive Or(1:w1336, 2:w1337) -> (0:w1342:bool)
          n463 = Build Array(w1337, w1336) -> (w1341:bool[])
          n464 = And(x=w1335, y=w1342) -> (x .and. y?=w1343:bool)
          n465 = Boolean Array To Number(Boolean array=w1341) -> (number=w1340:u32)
        }
        n466 = case shown="1, Default" w1275 {
          tunnel: [u16 3 u16 4] -> w1271
          tunnel: ["Condenser Merkava" "Condenser India"] -> w1274
          frame 1, Default {
          }
          frame 2 {
          }
        }
        "UUT" <- w1274
        n467 = property on="Pannel User Message" class="Str"(error in=w1272, "Value"="Tester initialization in process..." ("Pannel User Message")) -> (error out=w1295:errorcluster)  [unwired: 1 in, 1 out]
        n468 = call "ATRBuild.vi"("error constant"=w1295, "UUT In"=w1271) -> ("error constant 2"=w1306:errorcluster, "TestArray"=→"TestArray":string[], "TestArray Out"=w1305:string[][])  [unwired: 7 in]
        n469 = for {
          tunnel: w1305 -> [w1402] mode=indexing
          tunnel: w1306 -> [w1400]
          tunnel: [w1399] -> w1310
          tunnel: w1305 -> [w1398]
          i -> [w1401]
          n470 = for {
            tunnel: w1402 -> [_] mode=indexing
            tunnel: w1401 -> [w1408]
            tunnel: w1400 -> [w1405]
            tunnel: [w1404] -> w1399
            tunnel: w1398 -> [w1403]
            i -> [w1409]
            n471 = Bundle By Name(cluster=T10 {"Row"=0, "Column"=0} ("Active Cell:Active Cell"), "Row"=w1408, "Column"=w1409) -> (w1407:T10)
            n472 = control-ref of="ATR"() -> (w1406:refnum<vi>)
            n473 = property class="Tbl (strict)"(reference=w1406, error in=w1405, "Active Cell"=w1407, "Cell BG Color"=u32 16777226, "Value"=w1403) -> (error out=w1404:errorcluster)  [unwired: 1 out]
          }
        }
        n474 = call "DataFrom_ini (SubVI).vi"("error in (no error)"=w1310, "UUT"=w1274, "appended path"=w1312) -> ("error out"=w1281:errorcluster, "FileName"=w1300:string, "Next SN"=w1288:i32, "UUT SoftwareVer"=w1287:string, "ParamVersion"=→"ParamVersion":string, "PN"=w1285:string)  [unwired: 3 in]
        "UUT SoftwareVer" <- w1287
        "Next SN" <- w1288
        "FileName" <- w1300
        "PN" <- w1285
        n475 = Decrement(x=w1288) -> (x-1=w1289:i32)
        n476 = Number To Decimal String(number=w1289) -> (decimal integer string=w1286:string)  [unwired: 1 in]
        n477 = control-ref of="ATR"() -> (w1297:refnum<vi>)
        n478 = Build Array(w1287, w1287, w1286, w1285) -> (w1284:string[])
        n479 = call "Boards S/N"("error in (no error)"=w1281) -> ("POWER Board S/N"=→"POWER Board S/N":string, "DSP Board S/N"=→"DSP Board S/N":string, "error out"=w1280:errorcluster)  [unwired: 15 in, 1 out]
        n480 = for {
          tunnel: w1280 -> [w1350]
          tunnel: w1297 -> [w1348]
          tunnel: string[] ["RS232 Comm. + Version", "CAN Comm.", "Unit Serial number", "Unit Part number"] -> [w1347] mode=indexing
          tunnel: [w1346] -> w1298
          tunnel: w1284 -> [w1344] mode=indexing
          n481 = call "Find_Number_LineMARVIN.vi"("Test Paragraph"=w1347, "error in"=w1350, "TableIn"=w1348) -> ("error out"=w1349:errorcluster, "Line number"=w1345:i32)  [unwired: 2 in, 2 out]
          n482 = call "InsertSingleData.vi"("String In"=w1344, "error in (no error)"=w1349, "Col"=2, "Row"=w1345, "Table in"=w1348) -> ("error out"=w1346:errorcluster)  [unwired: 6 in]
        }
        n483 = control-ref of="This VI"() -> (w1296:refnum<vi>)
        n484 = call "COM UUT Board.vi"("error in (no error)"=w1298, "VI reference (current VI)"=w1296, "VISA resource name 2"=w1303) -> ("error out"=w1269:errorcluster, ".not. x?"=w1293:bool, "VISA resource name out"=w1266:refnum<visa-resource-name>)  [unwired: 6 in]
        "Serial Status" <- w1293
        n485 = call "RS232 DTR RTS.vi"("error in (no error)"=w1269, "Func"=enum16{"Init", "VEnable", "PowerOnOff"}."Init", "TesterCOM in"=w1266) -> ("error out"=w1265:errorcluster)  [unwired: 8 in]
        n486 = call "RS232 DTR RTS.vi"("error in (no error)"=w1265, "Func"=enum16{"Init", "VEnable", "PowerOnOff"}."PowerOnOff", "On/Off"=TRUE, "TesterCOM in"=w1266) -> ("error out"=w1264:errorcluster)  [unwired: 7 in]
        n487 = case shown="True" w1293 {
          tunnel: w1264 -> [w1352 w1375]
          tunnel: w1266 -> [w1353 w1374]
          tunnel: [w1353 w1365] -> w1276
          tunnel: [w1352 w1359] -> w1278
          tunnel: w1300 -> [_ w1358]
          tunnel: w1287 -> [_ w1354]
          frame False {
          }
          frame True {
            n488 = VISA Flush I/O Buffer(VISA resource name=w1374, error in (no error)=w1375) -> (VISA resource name out=w1365:refnum<visa-resource-name>, error out=w1373:errorcluster)  [unwired: 1 in]
            n489 = call "Display Message to User2"("error in (no error)"=w1373) -> ("error out"=w1372:errorcluster, "Yes"=w1371:bool)  [unwired: 9 in]
            n490 = case shown="True" w1371 {
              tunnel: w1372 -> [w1376 w1397]
              tunnel: [w1376 w1380] -> w1370
              tunnel: w1365 -> [_ w1395]
              tunnel: w1358 -> [_ w1388]
              frame False {
              }
              frame True {
                n491 = local read "TesterCOM"() -> (w1377:refnum<visa-resource-name>)
                n492 = call "SetParam.vi"("RS"=TRUE, "error in (no error)"=w1397, "Visa"=w1395, "Filein"=w1388) -> ("error out"=w1385:errorcluster)  [unwired: 7 in]
                n493 = call "RS232 DTR RTS.vi"("error in (no error)"=w1385, "Func"=enum16{"Init", "VEnable", "PowerOnOff"}."PowerOnOff", "On/Off"=FALSE, "TesterCOM in"=w1377) -> ("error out"=w1384:errorcluster)  [unwired: 7 in]
                n494 = control-ref of="Pannel User Message"() -> (w1394:refnum<vi>)
                n495 = control-ref of="Motor Speed RPM Serial"() -> (w1392:refnum<vi>)
                n496 = control-ref of="Stop Button"() -> (w1393:refnum<vi>)
                n497 = call "Write panel message Kinetics (SubVI).vi"(4:"rpm"=w1392, 5:"rpm"=FALSE ("rpm"), "PrintTime"=TRUE, "Stop"=w1393, "error in (no error)"=w1384, "Time to wait"=20.0, "Strin"="Restart the UUT\nPlease wait...", "String in"=w1394) -> ("error out"=w1382:errorcluster)  [unwired: 2 in, 1 out]
                n498 = call "RS232 DTR RTS.vi"("error in (no error)"=w1382, "Func"=enum16{"Init", "VEnable", "PowerOnOff"}."PowerOnOff", "On/Off"=TRUE, "TesterCOM in"=w1377) -> ("error out"=w1381:errorcluster)  [unwired: 7 in]
                n499 = call "Time Delay12"("error in (no error)"=w1381) -> ("error out"=w1380:errorcluster)  [unwired: 10 in]
              }
            }
            n500 = call "Serial.vi"("error in (no error)"=w1370, "write buffer"="SN\r\n", "VISA resource name"=w1365) -> ("error out"=w1366:errorcluster, "read buffer"=w1360:string)  [unwired: 7 in]
            n501 = property on="UUT SN Report" class="Str"("Value"=w1360) -> ()  [unwired: 2 in, 2 out]
            n502 = Decimal String To Number(string=w1360) -> (number=→"Current SN":i32)  [unwired: 2 in, 1 out]
            n503 = call "Serial.vi"("error in (no error)"=w1366, "write buffer"="VR\r\n", "VISA resource name"=w1365) -> ("error out"=w1361:errorcluster, "read buffer"=w1355:string)  [unwired: 7 in]
            n504 = control-ref of="ATR"() -> (w1362:refnum<vi>)
            n505 = call "Find_Number_LineMARVIN.vi"("Test Paragraph"="RS232 Comm. + Version", "TableIn"=w1362) -> ("Line number"=w1363:i32)  [unwired: 3 in, 3 out]
            n506 = Equal?(x=w1355, y=w1354) -> (x = y?=w1356:bool)
            n507 = call "PassOrFail (SubVI).vi"("String Res"=w1355, "index (row)"=w1363, "error in (no error)"=w1361, "Data in"=-3.0, "Pass?Fail"=w1356, "Table in"=w1362) -> ("error out"=w1359:errorcluster)  [unwired: 5 in]
          }
        }
        n508 = disable-structure shown="Enabled" {
          disable-tunnel: w1278 -> [w1324 w1330]
          disable-tunnel: [w1323 w1330] -> w1277
          disable-tunnel: w1276 -> [w1322 _]
          disable-tunnel: w1274 -> [w1321 _]
          frame Disabled {
            n509 = case shown="\"Condenser India\", \"Condenser Merkava\"" w1321 {
              tunnel: w1324 -> [w1325 w1328]
              tunnel: [w1325 w1327] -> w1323
              tunnel: w1322 -> [_ w1326]
              frame "False", Default {
              }
              frame "Condenser India", "Condenser Merkava" {
                n510 = call "Serial.vi"("error in (no error)"=w1328, "write buffer"="EP=1\r\nVC=1000\r\n", "VISA resource name"=w1326) -> ("error out"=w1327:errorcluster)  [unwired: 7 in, 1 out]
              }
            }
          }
          frame Enabled {
          }
        }
        n511 = property on="TesterCOM" class="VISAName"("Value"=w1266) -> ()  [unwired: 2 in, 2 out]
        n512 = property on="Pannel User Message" class="Str"(error in=w1277, "Value"="You can press start to execute(s) test(s)." ("Pannel User Message")) -> (error out=w1292:errorcluster)  [unwired: 1 in, 1 out]
        n513 = property on="Start" class="Bool (strict)"(error in=w1292, "DisabledEnum"=w1311) -> (error out=w1302:errorcluster)  [unwired: 1 in, 1 out]
        n514 = property on="Report" class="Bool (strict)"(error in=w1302, "DisabledEnum"=w1311) -> (error out=w1301:errorcluster)  [unwired: 1 in, 1 out]
      }
      frame "Stop" {
        w1433 = 0
        n515 = control-ref of="ATR"() -> (w1432:refnum<vi>)
        n516 = call "PassFailUUT (SubVI).vi"("error in (no error)"=w1418, "Table in"=w1432) -> ("PassFaileUUTresult"=w1425:bool)  [unwired: 7 in, 2 out]
        n517 = property on="Test Failed" class="Bool (strict)"("Value"=w1425) -> ()  [unwired: 2 in, 2 out]
        n518 = flat-sequence {
          tunnel: w1418 -> [w1477]
          tunnel: [w1476] -> w1453
          frame #0 {
            n519 = control-ref of="Pannel User Message"() -> (w1479:refnum<vi>)
            n520 = property class="Str"(reference=w1479, error in=w1477, "Value"="Program Stopped...\r\nPlease turn OFF All Power sinks") -> (error out=w1476:errorcluster)  [unwired: 1 out]
          }
        }
        n521 = Select(t="PASS" ("name or relative path"), s=w1425, f="FAIL" ("name or relative path")) -> (s? t:f=w1424:string)
        n522 = call <vilib>:"Application Directory.vi"() -> ("Application Directory"=w1428:path)
        n523 = Build Path(base path=w1428, name or relative path="data\\TestResult.ini") -> (appended path=w1431:path)
        n524 = call <vilib>:"Open Config Data.vi"("configuration file path"=w1431) -> ("error out"=w1429:errorcluster, "refnum"=w1430:T3)  [unwired: 2 in, 7 out]
        n525 = call-poly <vilib>:"Write Key.vi"("section"="Kinetics", "error in (no error)"=w1429, "value"=w1424, "key"="Result", "refnum"=w1430) -> ("error out"=w1427:errorcluster, "refnum out"=w1426:T3)  [unwired: 4 in, 1 out]
        n526 = call <vilib>:"Close Config Data.vi"("error in (no error)"=w1427, "refnum"=w1426) -> ()  [unwired: 8 in, 2 out]
        n527 = property on="VISA Current" class="VISAName"() -> ("Value"=w1415:refnum<visa-resource-name>)  [unwired: 2 in, 2 out]
        n528 = local read "TesterCOM"() -> (w1413:refnum<visa-resource-name>)
        n529 = VISA Close(VISA resource name=w1460, error in (no error)=w1453) -> (error out=w1455:errorcluster)
        n530 = VISA Close(VISA resource name=w1415) -> (error out=w1414:errorcluster)  [unwired: 1 in]
        n531 = property on="Stop Button" class="Bool (strict)"() -> ("Value"=w1436:bool)  [unwired: 2 in, 2 out]
        n532 = call "RS232 DTR RTS.vi"("Func"=enum16{"Init", "VEnable", "PowerOnOff"}."Init", "On/Off"=FALSE, "TesterCOM in"=w1413) -> ("error out"=w1416:errorcluster)  [unwired: 8 in]
        n533 = property on="ClosePanel" class="Bool (strict)"() -> ("Value"=w1437:bool)  [unwired: 2 in, 2 out]
        n534 = Or(x=w1437, y=w1436) -> (x .or. y?=w1435:bool)
        n535 = Flush Queue(queue=w1456, error in (no error)=w1455) -> (queue out=w1458:refnum<queue>, error out=w1457:errorcluster)  [unwired: 1 out]
        n536 = case shown="True" w1435 {
          tunnel: w1458 -> [w1462 w1463]
          tunnel: w1457 -> [w1461 w1465]
          tunnel: [w1461 w1464] -> w1449
          tunnel: [w1462 w1463] -> w1434
          frame False {
          }
          frame True {
            n537 = Release Queue(queue=w1463, error in (no error)=w1465) -> (error out=w1464:errorcluster)  [unwired: 1 in, 2 out]
          }
        }
        n538 = Merge Errors(w1449, w1453, w1416, w1414) -> (w1448:errorcluster)
        n539 = property on="Refresh Button" class="Bool (strict)"() -> ("Value"=w1438:bool)  [unwired: 2 in, 2 out]
        n540 = call <vilib>:"Clear Errors.vi"("error in (no error)"=w1448) -> ("error out"=w1447:errorcluster)  [unwired: 5 in, 1 out]
        n541 = property on="Stop Button" class="Bool (strict)"() -> ("Value"=w1442:bool)  [unwired: 2 in, 2 out]
        n542 = property on="ClosePanel" class="Bool (strict)"(error in=w1447) -> (error out=w1445:errorcluster, "Value"=w1446:bool)  [unwired: 1 in, 1 out]
        n543 = Not(x=w1438) -> (.not. x?=w1439:bool)
        n544 = Select(t=T2."Initialize", s=w1438, f=T2."Stop") -> (s? t:f=w1450:T2)
        n545 = Not(x=w1442) -> (.not. x?=w1441:bool)
        n546 = Compound Arithmetic op=AND(w1446, w1441, w1439) -> (w1443:bool)
        n547 = case shown="False" w1443 {
          tunnel: w1445 -> [w1468 w1472]
          tunnel: [w1468 w1472] -> w1444
          tunnel: [w1467 w1471] -> w1440
          tunnel: w1438 -> [w1466 _]
          frame False {
            n548 = case shown="False" w1466 {
              tunnel: [TRUE FALSE] -> w1467
              frame False {
              }
              frame True {
              }
            }
          }
          frame True {
            n549 = flat-sequence {
              tunnel: [TRUE] -> w1471
              frame #0 {
              }
              frame #1 {
                n550 = control-ref of="This VI"() -> (w1475:refnum<vi>)
                n551 = property class="VI"(reference=w1475, "FP.State"=T11."Closed" ("Front Panel Window:State")) -> ()  [unwired: 1 in, 2 out]
              }
            }
          }
        }
      }
      frame "MainProgram" {
        n552 = event shown="[6] \"Start\": Value Change" {
          selector: w1490 -> [_ _ _ _ _ _ _ _ _ _ _ _ _]
          dyn-events: _ -> [_ _ _ _ _ _ _ _ _ _ _ _ _]
          timeout: "EventTimeout" -> [_ _ _ _ _ _ _ _ _ _ _ _ _]
          tunnel: [T2."MainProgram" T2."MainProgram" T2."MainProgram" T2."MainProgram" T2."MainProgram" T2."Stop" T2."MainProgram" w1778 T2."MainProgram" T2."MainProgram" T2."MainProgram" T2."Stop" T2."MainProgram"] -> w1499
          tunnel: [w1512 w1551 w1615 w1622 w1631 w1649 w1665 w1822 w1883 w1896 _ w1914 w1915] -> w1493
          tunnel: w1497 -> [w1512 w1551 w1614 w1624 w1631 w1649 _ w1822 w1884 w1895 w1903 w1914 w1915]
          tunnel: [w1510 w1545 w1616 w1623 w1632 w1647 w1658 w1783 w1881 w1893 _ w1912 w1918] -> w1494
          tunnel: w1495 -> [w1510 w1545 w1616 w1623 w1632 w1647 w1658 w1783 w1881 w1893 _ w1912 w1918]
          tunnel: w1492 -> [w1514 w1555 w1611 w1620 w1629 w1646 w1666 w1806 w1880 w1892 w1905 w1911 w1920]
          tunnel: [w1514 w1555 w1611 w1620 w1629 w1646 w1664 w1806 w1880 w1892 w1905 w1911 w1920] -> w1491
          tunnel: w1489 -> [_ _ _ _ _ _ _ w1761 _ _ _ _ _]
          tunnel: w1488 -> [w1515 w1554 w1610 w1619 w1628 w1644 w1662 w1787 w1879 w1891 w1904 w1910 w1919]
          tunnel: [w1515 w1554 w1610 w1619 w1628 w1644 w1662 w1786 w1879 w1891 w1904 w1910 w1919] -> w1487
          tunnel: w1486 -> [_ w1552 _ _ _ _ _ w1785 _ _ _ _ _]
          tunnel: w1485 -> [_ w1544 _ _ _ _ _ _ _ _ _ _ _]
          tunnel: w1484 -> [_ _ _ _ _ _ _ _ w1878 _ _ _ _]
          tunnel: w1483 -> [_ w1533 w1609 w1618 w1627 w1641 w1661 w1762 w1876 w1890 w1901 w1909 w1917]
          tunnel: [_ w1533 w1609 w1618 w1627 w1641 w1661 w1762 w1876 w1890 w1901 w1909 w1917] -> w1482
          tunnel: w1481 -> [w1511 w1532 w1608 w1617 w1626 w1640 w1660 w1754 w1875 w1889 w1900 w1908 w1916]
          tunnel: [w1511 w1532 w1608 w1617 w1626 w1640 w1660 w1754 w1875 w1889 w1900 w1908 w1916] -> w1480
          event Timeout {
            n553 = event-data() -> ()  [unwired: 1 in, 3 out]
            n554 = property on="ClosePanel" class="Bool (strict)"("Value"=FALSE ("ClosePanel")) -> ()  [unwired: 2 in, 2 out]
            n555 = property on="VISA Current" class="VISAName"() -> ("Value"=w1502:refnum<visa-resource-name>)  [unwired: 2 in, 2 out]
            n556 = Not Equal?(x=w1502, y=refnum<visa-resource-name> "COMx") -> (x != y?=w1503:bool)
            n557 = case shown="True" w1503 {
              tunnel: w1502 -> [_ w1521]
              frame False {
              }
              frame True {
                n558 = call "ReadCurrent.vi"("LoopFromMain"=TRUE, "VISA resource name"=w1521) -> ("CurrentSens"=→"CurrentSens":bool, "CurrentOut"=w1519:string)  [unwired: 7 in, 1 out]
                "Current" <- w1519
                n559 = Fract/Exp String To Number(string=w1519) -> (number=→"CurrentOut":dbl)  [unwired: 3 in, 1 out]
              }
            }
            n560 = Not Equal?(x=w1510, y=refnum<visa-resource-name> "COMx") -> (x != y?=w1508:bool)
            n561 = control-ref of="ATR"() -> (w1500:refnum<vi>)
            n562 = call "PassFailUUT (SubVI).vi"("Table in"=w1500) -> ("PassFaileUUTresult"=w1501:bool)  [unwired: 8 in, 2 out]
            n563 = case shown="True" w1508 {
              tunnel: w1510 -> [_ w1527]
              frame False {
              }
              frame True {
                n564 = call "Serial.vi"("Clear Log"=FALSE, "write buffer"="VC\r\n", "VISA resource name"=w1527) -> ("read buffer"=w1523:string)  [unwired: 7 in, 1 out]
                n565 = Fract/Exp String To Number(string=w1523) -> (number=→"Motor Speed RPM Serial":dbl)  [unwired: 3 in, 1 out]
              }
            }
            n566 = property on="Test Failed" class="Bool (strict)"("Value"=w1501) -> ()  [unwired: 2 in, 2 out]
            n567 = property on="Automation" class="Bool (strict)"() -> ("Value"=w1507:bool)  [unwired: 2 in, 2 out]
            n568 = property on="Start" class="Bool (strict)"() -> ("Value"=w1505:bool)  [unwired: 2 in, 2 out]
            n569 = Or(x=w1507, y=w1505) -> (x .or. y?=w1506:bool)
            n570 = case shown="False" w1506 {
              frame False {
                n571 = property on="Pannel User Message" class="Str"("Value"="You can press start to execute(s) test(s).") -> ()  [unwired: 2 in, 2 out]
              }
              frame True {
              }
            }
          }
          event "SetSN": Value Change {
            n572 = event-data() -> ()  [unwired: 1 in, 6 out]
            n573 = property on="UUT" class="Str"() -> ("Value"=w1531:string)  [unwired: 2 in, 2 out]
            n574 = case shown="\"BLDC 30A\", Default" w1531 {
              tunnel: [26 26 26 26 35] -> w1529
              frame "BLDC 30A", Default {
              }
              frame "Warrior 60A" {
              }
              frame "Condenser Merkava" {
              }
              frame "Condenser India" {
              }
              frame "BLDC 60A" {
              }
            }
            n575 = control-ref of="ATR"() -> (w1536:refnum<vi>)
            n576 = property on="Current SN" class="DigNum (strict)"(error in=w1551) -> (error out=w1535:errorcluster, "Value"=w1550:i32)  [unwired: 1 in, 1 out]
            n577 = call "PassFailUUT (SubVI).vi"("error in (no error)"=w1535, "Table in"=w1536) -> ("Total Pass"=w1530:u8)  [unwired: 7 in, 2 out]
            n578 = Equal To 0?(x=w1550) -> (x = 0?=w1547:bool)
            n579 = Equal?(x=w1550, y=-1) -> (x = y?=w1548:bool)
            n580 = Equal?(x=w1530, y=w1529) -> (x = y?=w1528:bool)
            n581 = Or(x=w1548, y=w1547) -> (x .or. y?=w1546:bool)
            n582 = property on="Tester Status" class="Bool (strict)"() -> ("Value"=w1537:bool)  [unwired: 2 in, 2 out]
            n583 = property on="Serial Status" class="Bool (strict)"() -> ("Value"=w1542:bool)  [unwired: 2 in, 2 out]
            n584 = And(x=w1542, y=w1537) -> (x .and. y?=w1538:bool)
            n585 = case shown="True" w1538 {
              tunnel: w1552 -> [_ w1574]
              tunnel: w1546 -> [_ w1563]
              tunnel: w1545 -> [_ w1573]
              tunnel: w1544 -> [_ w1572]
              tunnel: [errorcluster {"status"=FALSE, "code"=0, "source"=""} ("error out") w1571] -> w1541
              tunnel: [w1561 w1570] -> w1543
              tunnel: w1528 -> [_ w1564]
              frame False {
                w1561 = FALSE ("Value")
                n586 = property on="SetSN" class="Bool (strict)"("Value"=w1561) -> ()  [unwired: 2 in, 2 out]
                n587 = call "Display Message to User10"() -> ()  [unwired: 10 in, 2 out]
              }
              frame True {
                n588 = property on="Test Failed" class="Bool (strict)"() -> ("Value"=w1568:bool)  [unwired: 2 in, 2 out]
                n589 = property on="Automation" class="Bool (strict)"() -> ("Value"=w1570:bool)  [unwired: 2 in, 2 out]
                n590 = Not(x=w1568) -> (.not. x?=w1569:bool)
                n591 = Select(t=w1569, s=w1570, f=w1572) -> (s? t:f=w1566:bool)
                n592 = Or(x=w1564, y=w1566) -> (x .or. y?=w1565:bool)
                n593 = And(x=w1563, y=w1565) -> (x .and. y?=w1567:bool)
                n594 = case shown="True" w1567 {
                  tunnel: w1574 -> [_ w1605]
                  tunnel: w1573 -> [_ w1598]
                  tunnel: [w1576 w1590] -> w1571
                  tunnel: w1563 -> [w1575 _]
                  frame False {
                    n595 = case shown="True" w1575 {
                      tunnel: [w1578 w1579] -> w1576
                      frame False {
                        n596 = call "Display Message to User9"() -> ("error out"=w1578:errorcluster)  [unwired: 10 in, 1 out]
                      }
                      frame True {
                        n597 = call "Display Message to User3"() -> ("error out"=w1579:errorcluster)  [unwired: 10 in, 1 out]
                      }
                    }
                    n598 = property on="Automation" class="Bool (strict)"(error in=w1576, "Value"=FALSE ("Automation")) -> ()  [unwired: 1 in, 2 out]
                  }
                  frame True {
                    w1597 = FALSE ("SetSN")
                    n599 = property on="Next SN" class="DigNum (strict)"() -> ("Value"=w1585:i32)  [unwired: 2 in, 2 out]
                    n600 = local read "TesterCOM"() -> (w1581:refnum<visa-resource-name>)
                    n601 = call "RS232 DTR RTS.vi"("Func"=enum16{"Init", "VEnable", "PowerOnOff"}."VEnable", "On/Off"=FALSE, "TesterCOM in"=w1581) -> ("error out"=w1587:errorcluster)  [unwired: 8 in]
                    n602 = call <vilib>:"Clear Errors.vi"("error in (no error)"=w1587) -> ("error out"=w1588:errorcluster)  [unwired: 5 in, 1 out]
                    n603 = Number To Decimal String(number=w1585) -> (decimal integer string=w1586:string)  [unwired: 1 in]
                    "UUT SN Report" <- w1586
                    n604 = Search and Replace String(input string="EP=1\r\nSN=0\r\n" ("write buffer"), search string="0", replace string=w1586) -> (result string=w1600:string)  [unwired: 5 in, 3 out]
                    n605 = call "Serial.vi"("error in (no error)"=w1588, "Clear Log"=FALSE, "write buffer"=w1600, "VISA resource name"=w1598) -> ("error out"=w1584:errorcluster)  [unwired: 6 in, 1 out]
                    n606 = property on="UUT" class="Str"(error in=w1584) -> ("Value"=w1583:string)  [unwired: 1 in, 2 out]
                    n607 = call <vilib>:"Open Config Data.vi"("create file if necessary (T)"=FALSE, "configuration file path"=w1605) -> ("error out"=w1603:errorcluster, "refnum"=w1604:T3)  [unwired: 1 in, 7 out]
                    n608 = call-poly <vilib>:"Write Key.vi"("section"=w1583, "error in (no error)"=w1603, "value"=w1586, "key"="SN", "refnum"=w1604) -> ("error out"=w1593:errorcluster, "refnum out"=w1592:T3)  [unwired: 4 in, 1 out]
                    n609 = call <vilib>:"Close Config Data.vi"("error in (no error)"=w1593, "refnum"=w1592) -> ("error out"=w1591:errorcluster)  [unwired: 8 in, 1 out]
                    n610 = property on="Current SN" class="DigNum (strict)"("Value"=w1585) -> ()  [unwired: 2 in, 2 out]
                    n611 = property on="SetSN" class="Bool (strict)"(error in=w1591, "Value"=w1597) -> (error out=w1596:errorcluster)  [unwired: 1 in, 1 out]
                    n612 = property on="Automation" class="Bool (strict)"(error in=w1596, "Value"=w1597) -> (error out=w1595:errorcluster)  [unwired: 1 in, 1 out]
                    n613 = Increment(x=w1585) -> (x+1=w1594:i32)
                    n614 = property on="Next SN" class="DigNum (strict)"(error in=w1595, "Value"=w1594) -> (error out=w1590:errorcluster)  [unwired: 1 in, 1 out]
                  }
                }
              }
            }
            n615 = call <vilib>:"Clear Errors.vi"("error in (no error)"=w1541) -> ("error out"=w1534:errorcluster)  [unwired: 5 in, 1 out]
            n616 = property on="SetSN" class="Bool (strict)"(error in=w1534, "Value"=FALSE ("SetSN")) -> (error out=w1540:errorcluster)  [unwired: 1 in, 1 out]
            n617 = case shown="True" w1543 {
              tunnel: w1540 -> [_ _]
              frame False {
              }
              frame True {
                w1607 = TRUE ("Value (Signaling)")
                n618 = property on="Report" class="Bool (strict)"("Val(Sgnl)"=w1607, "Value"=w1607) -> ()  [unwired: 2 in, 2 out]
              }
            }
          }
          event "ATR": Mouse Enter {
            n619 = event-data() -> ()  [unwired: 1 in, 4 out]
            n620 = call-poly <vilib>:"Set Cursor.vi"("error in (no error)"=w1614, "icon"=u16 1) -> ("error out"=w1615:errorcluster)  [unwired: 8 in, 1 out]
          }
          event "ATR": Mouse Leave {
            n621 = event-data() -> ()  [unwired: 1 in, 4 out]
            n622 = call-poly <vilib>:"Set Cursor.vi"("error in (no error)"=w1624, "icon"=u16 0) -> ("error out"=w1622:errorcluster)  [unwired: 8 in, 1 out]
          }
          event "ATR": Mouse Down? {
            n623 = event-data() -> ("Coords"=w1639:T13)  [unwired: 1 in, 4 out]
            n624 = invoke on="ATR" class="Tbl (strict)" method="Point To Row Column"("Point"=w1639) -> ("InBounds"=w1635:bool, "CellPosition"=w1634:T10)  [unwired: 5 in, 4 out]
            n625 = Greater Than 0?(x=w1634) -> (x > 0?=w1638:cluster{"Row":bool, "Column":bool})
            n626 = Cluster To Array(cluster=w1638) -> (array=w1637:bool[])
            n627 = Or Array Elements(Boolean array=w1637) -> (logical OR=w1636:bool)
            n628 = Or(x=w1635, y=w1636) -> (x .or. y?=w1633:bool)
            n629 = event-data("Discard?"=w1633) -> ()  [unwired: 1 in, 1 out]
          }
          event Panel Close? {
            n630 = event-data() -> ("VIRef"=w1645:refnum<vi>)  [unwired: 1 in, 3 out]
            n631 = Close Reference(reference=w1645) -> ()  [unwired: 1 in, 1 out]
            n632 = disable-structure shown="Disabled" {
              frame Disabled {
                n633 = property on="Stop Button" class="Bool (strict)"("Val(Sgnl)"=TRUE ("Stop Button"), "Value"=FALSE ("Stop Button")) -> ()  [unwired: 2 in, 2 out]
              }
              frame Enabled {
              }
            }
            n634 = event-data("Discard?"=TRUE) -> ()  [unwired: 1 in, 1 out]
            "ClosePanel" <- TRUE ("ClosePanel")
          }
          event "Start": Value Change {
            w1656 = string[] []  # TestArray
            n635 = event-data() -> ()  [unwired: 1 in, 2 out]
            n636 = while {
              tunnel: [w1680] -> w1655
              tunnel: [w1679] -> w1653
              shift-right: [w1677] -> _
              shift-left: enum16{"Stop", "Tests", "Bit test", "Start"}."Start" -> [w1678]
              tunnel: w1656 -> [w1676]
              stop <- w1675 stop-if-true
              n637 = case shown="\"Tests\"" w1678 {
                tunnel: [w1685 w1690 w1700 w1712] -> w1680
                tunnel: [errorcluster {"status"=FALSE, "code"=0, "source"=""} ("error out") w1689 errorcluster {"status"=FALSE, "code"=0, "source"=""} ("error out") w1710] -> w1679
                tunnel: [w1684 w1696 enum16{"Stop", "Tests", "Bit test", "Start"}."Stop" w1706] -> w1677
                tunnel: w1676 -> [w1685 _ w1700 w1712]
                tunnel: [w1683 w1695 FALSE FALSE] -> w1675
                frame "Stop", Default {
                  n638 = flat-sequence {
                    tunnel: [enum16{"Stop", "Tests", "Bit test", "Start"}."Stop"] -> w1684
                    tunnel: [TRUE] -> w1683
                    frame #0 {
                    }
                  }
                  n639 = property on="Start" class="Bool (strict)"("Value"=FALSE ("Start")) -> ()  [unwired: 2 in, 2 out]
                }
                frame "Tests" {
                  w1694 = T9."Disabled and Grayed Out" ("Disabled")
                  n640 = property on="TestArray" class="Arr (strict)"() -> (error out=w1689:errorcluster, "Value"=w1691:string[])  [unwired: 2 in, 1 out]
                  n641 = call "Start Test Selection (SubVI).vi"("TestArrayIn"=w1691) -> ("AutoOut"=w1688:bool, "TestArrayOut"=w1690:string[])  [unwired: 9 in]
                  "Automation" <- w1688
                  n642 = property on="Start" class="Bool (strict)"("DisabledEnum"=w1694) -> ()  [unwired: 2 in, 2 out]
                  n643 = property on="Report" class="Bool (strict)"("DisabledEnum"=w1694) -> ()  [unwired: 2 in, 2 out]
                  n644 = control-ref of="ATR"() -> (w1692:refnum<vi>)
                  n645 = property on="Stop Button" class="Bool (strict)"("Value"=FALSE ("Stop Burn-in")) -> ()  [unwired: 2 in, 2 out]
                  n646 = case shown="True" w1688 {
                    tunnel: w1692 -> [_ w1697]
                    frame False {
                    }
                    frame True {
                      n647 = call "ResetTable Result (SubVI).vi"("Table in"=w1697) -> ()  [unwired: 11 in]
                    }
                  }
                  n648 = flat-sequence {
                    tunnel: [enum16{"Stop", "Tests", "Bit test", "Start"}."Tests"] -> w1696
                    tunnel: [TRUE] -> w1695
                    frame #0 {
                    }
                  }
                }
                frame "Bit test" {
                }
                frame "Start" {
                  n649 = property on="Tester Status" class="Bool (strict)"() -> (error out=w1709:errorcluster, "Value"=w1708:bool)  [unwired: 2 in, 1 out]
                  n650 = property on="CurrentSens" class="Bool (strict)"() -> ("Value"=w1704:bool)  [unwired: 2 in, 2 out]
                  n651 = property on="Serial Status" class="Bool (strict)"(error in=w1709) -> ("Value"=w1707:bool)  [unwired: 1 in, 2 out]
                  n652 = And(x=w1708, y=w1707) -> (x .and. y?=w1705:bool)
                  n653 = case shown="True" w1705 {
                    tunnel: [w1714 w1717] -> w1710
                    tunnel: [enum16{"Stop", "Tests", "Bit test", "Start"}."Stop" w1716] -> w1706
                    tunnel: w1704 -> [_ w1715]
                    frame False {
                      n654 = call "Display Message to User5"() -> ("error out"=w1714:errorcluster)  [unwired: 10 in, 1 out]
                    }
                    frame True {
                      n655 = case shown="True" w1715 {
                        tunnel: [w1718 w1724] -> w1717
                        tunnel: [enum16{"Stop", "Tests", "Bit test", "Start"}."Stop" enum16{"Stop", "Tests", "Bit test", "Start"}."Tests"] -> w1716
                        frame False {
                          n656 = call "Display Message to User"() -> ("error out"=w1718:errorcluster)  [unwired: 10 in, 1 out]
                        }
                        frame True {
                          n657 = control-ref of="Motor Speed RPM Serial"() -> (w1721:refnum<vi>)
                          n658 = control-ref of="Stop Button"() -> (w1722:refnum<vi>)
                          n659 = control-ref of="Pannel User Message"() -> (w1723:refnum<vi>)
                          n660 = call "Write panel message Kinetics (SubVI).vi"(4:"rpm"=w1721, 5:"rpm"=FALSE ("rpm"), "PrintTime"=FALSE, "Stop"=w1722, "Time to wait"=0.0, "Strin"="TESTER BIT TEST OPERATION IN PROCESS\nPlease wait...", "String in"=w1723) -> ("error out"=w1724:errorcluster)  [unwired: 3 in, 1 out]
                        }
                      }
                    }
                  }
                }
              }
            }
            n661 = Array Size(array=w1655) -> (size(s)=w1654:i32)
            n662 = case shown="1, Default" w1654 {
              tunnel: w1653 -> [w1668 w1672]
              tunnel: [w1668 w1671] -> w1652
              frame 0 {
              }
              frame 1, Default {
                n663 = local read "TesterCOM"() -> (w1670:refnum<visa-resource-name>)
                n664 = call "RS232 DTR RTS.vi"("error in (no error)"=w1672, "Func"=enum16{"Init", "VEnable", "PowerOnOff"}."PowerOnOff", "On/Off"=TRUE, "TesterCOM in"=w1670) -> ("error out"=w1673:errorcluster)  [unwired: 7 in]
                n665 = call "Time Delay"("error in (no error)"=w1673) -> ("error out"=w1671:errorcluster)  [unwired: 10 in]
              }
            }
            n666 = Bundle By Name(cluster=T1 {"VISA"="COM1", "TestArray"=[]}, "VISA"=w1658, "TestArray"=w1655) -> (w1659:T1)
            n667 = Enqueue Element(queue=w1666, element=w1659, error in (no error)=w1652) -> (queue out=w1664:refnum<queue>, error out=w1665:errorcluster)  [unwired: 2 out]
          }
          event "Report", "Stop Button": Value Change {
            w1764 = T14 1 items=["User Home"=0, "User Desktop"=1, "User Documents"=2, "User Application Data"=3, "User Preferences"=4, "User Temporary"=5, "Public Documents"=6, "Public Application Data"=7, "Public Preferences"=8, "Public Cache"=13, "System Core Libraries"=9, "System Installed Libraries"=10, "Application Files"=11, "Boot Volume Root"=12] ("system directory type")
            w1732 = FALSE ("Report")
            n668 = event-data() -> ("CtlRef"=w1782:refnum<vi>)  [unwired: 1 in]
            n669 = local read "UUT"() -> (w1729:string)
            n670 = call <vilib>:"Get System Directory.vi"("create directory if not found? (F)"=TRUE, "system directory type"=w1764) -> ("system directory"=w1763:path)  [unwired: 9 in]
            n671 = Build Path(base path=w1763, name or relative path="KineticsReports") -> (appended path=w1815:path)
            n672 = property on="Tester Status" class="Bool (strict)"() -> ("Value"=w1767:bool)  [unwired: 2 in, 2 out]
            n673 = property on="Serial Status" class="Bool (strict)"() -> ("Value"=w1768:bool)  [unwired: 2 in, 2 out]
            n674 = call <vilib>:"Check if File or Folder Exists.vi"("path"=w1815) -> ("error out"=w1813:errorcluster, "file or folder exists?"=w1816:bool, "dup path"=w1814:path)  [unwired: 8 in]
            n675 = To Upper Case(1:w1729) -> (0:w1730:string)
            n676 = And(x=w1768, y=w1767) -> (x .and. y?=w1769:bool)
            n677 = case shown="False" w1816 {
              tunnel: w1813 -> [w1872 w1873]
              tunnel: w1814 -> [w1871 w1874]
              tunnel: [w1870 w1874] -> w1766
              tunnel: [w1869 w1873] -> w1818
              frame False {
                n678 = Create Folder(path (use dialog)=w1871, error in=w1872) -> (created path=w1870:path, error out=w1869:errorcluster)  [unwired: 1 in, 1 out]
              }
              frame True {
              }
            }
            n679 = case shown="True" w1769 {
              tunnel: [w1823 "" ("read buffer")] -> w1804
              tunnel: [w1823 w1825] -> w1757
              tunnel: w1783 -> [_ w1833]
              tunnel: [w1823 w1842] -> w1760
              tunnel: [w1823 w1826] -> w1758
              tunnel: [w1823 "" ("read buffer")] -> w1776
              frame False {
                w1823 = "N_A" ("read buffer")
              }
              frame True {
                n680 = call "Serial.vi"("write buffer"="SN\r\n", "VISA resource name"=w1833) -> ("error out"=w1838:errorcluster, "read buffer"=w1840:string)  [unwired: 8 in]
                n681 = Decimal String To Number(string=w1840) -> (number=w1839:i32)  [unwired: 2 in, 1 out]
                n682 = Number To Decimal String(number=w1839, width (-)=i16 4) -> (decimal integer string=w1842:string)
                n683 = call "Serial.vi"("error in (no error)"=w1838, "write buffer"="VR\r\n", "VISA resource name"=w1833) -> ("error out"=w1834:errorcluster, "read buffer"=w1826:string)  [unwired: 7 in]
                n684 = call "Serial.vi"("error in (no error)"=w1834, "write buffer"="PN\r\n", "VISA resource name"=w1833) -> ("read buffer"=w1824:string)  [unwired: 7 in, 1 out]
                n685 = String Length(string=w1824) -> (length=w1831:i32)
                n686 = Subtract(x=6, y=w1831) -> (x-y=w1830:i32)
                n687 = for {
                  N: w1830 -> [_]
                  shift-right: [w1847] -> w1827
                  shift-left: "" -> [w1846]
                  n688 = Concatenate Strings(w1846, "0" ("string")) -> (w1847:string)
                }
                n689 = Concatenate Strings("RD" ("string"), w1827, w1824) -> (w1825:string)
              }
            }
            n690 = Get Date/Time String(want seconds? (F)=TRUE) -> (date string=w1817:string)  [unwired: 2 in, 1 out]
            n691 = call <vilib>:"Open Config Data.vi"("create file if necessary (T)"=FALSE, "configuration file path"=w1785) -> ("refnum"=w1795:T3)  [unwired: 1 in, 8 out]
            n692 = property on="Logger Path" class="Path"(error in=w1818, "Value"=w1766, "StartPath"=w1766) -> (error out=w1798:errorcluster)  [unwired: 1 in, 1 out]
            n693 = Search and Replace String(replace all?=TRUE ("replace all? (F)"), input string=w1817, search string="/") -> (result string=w1801:string)  [unwired: 5 in, 3 out]
            n694 = call-poly <vilib>:"Read Key.vi"("section"=w1729, "key"="version", "refnum"=w1795) -> ("error out"=w1790:errorcluster, "value"=w1793:string, "refnum out"=w1792:T3)  [unwired: 5 in, 1 out]
            n695 = call-poly <vilib>:"Read Key.vi"("section"="Kinetics", "error in (no error)"=w1790, "key"="Condenser Tester Software Ver", "refnum"=w1792) -> ("error out"=w1788:errorcluster, "value"=w1759:string, "refnum out"=w1791:T3)  [unwired: 4 in, 1 out]
            n696 = property on="POWER Board S/N" class="Str"() -> ("Value"=w1737:string)  [unwired: 2 in, 2 out]
            n697 = Concatenate Strings("ATR" ("string"), w1804, w1760, "_", w1801, ".docx" ("string")) -> (w1799:string)
            n698 = call <vilib>:"Close Config Data.vi"("error in (no error)"=w1788, "refnum"=w1791) -> ()  [unwired: 8 in, 2 out]
            n699 = Build Path(base path=w1766, name or relative path=w1799) -> (appended path=w1800:path)
            n700 = property on="DSP Board S/N" class="Str"() -> ("Value"=w1736:string)  [unwired: 2 in, 2 out]
            n701 = Concatenate Strings("  Rev-" ("string"), w1793) -> (w1784:string)
            n702 = while {
              tunnel: w1799 -> [w1854]
              tunnel: w1766 -> [w1851]
              shift-right: [w1853] -> w1797
              shift-left: w1800 -> [w1852]
              shift-right: [w1849] -> w1786
              shift-left: w1787 -> [w1850]
              tunnel: w1798 -> [w1855]
              tunnel: [w1856] -> w1765
              stop <- w1848 continue-if-true
              n703 = call <vilib>:"Check if File or Folder Exists.vi"("error in (no error)"=w1855, "path"=w1852) -> ("error out"=w1856:errorcluster, "file or folder exists?"=w1848:bool)  [unwired: 7 in, 1 out]
              n704 = case shown="True" w1848 {
                tunnel: w1854 -> [_ w1868]
                tunnel: w1850 -> [_ w1860]
                tunnel: [w1858 w1865] -> w1853
                tunnel: w1852 -> [w1858 _]
                tunnel: w1851 -> [_ w1866]
                tunnel: [1 w1859] -> w1849
                frame False {
                }
                frame True {
                  w1861 = ".docx" ("search string")
                  n705 = Search and Replace String(input string=w1868, search string=w1861) -> (result string=w1867:string)  [unwired: 6 in, 3 out]
                  n706 = Number To Decimal String(number=w1860) -> (decimal integer string=w1863:string)  [unwired: 1 in]
                  n707 = call <vilib>:"Space Constant.vi"() -> ("String"=w1862:string)
                  n708 = Concatenate Strings(w1867, w1862, w1863, w1861) -> (w1864:string)
                  n709 = Build Path(base path=w1866, name or relative path=w1864) -> (appended path=w1865:path)
                  n710 = Increment(x=w1860) -> (x+1=w1859:i32)
                }
              }
            }
            n711 = property on="ParamVersion" class="Str"() -> ("Value"=w1735:string)  [unwired: 2 in, 2 out]
            n712 = call "HeaderBis.vi"("UUTHeader"=w1730, "POWER SN"=w1737, "Revision Param"=w1735, "P/N UUT"=w1757, "DSP SN"=w1736, "Driver S/N"=w1760, "VR"=w1758, "Oper."=w1761, "Tester Software Ver"=w1759) -> ("table header"=w1756:string, "Array"=w1755:string[][])  [unwired: 4 in, 1 out]
            n713 = Open/Create/Replace File(file path (use dialog)=w1797, error in=w1765, operation (0:open)=T12."create") -> (error out=w1808:errorcluster)  [unwired: 3 in, 2 out]
            n714 = control-ref of="ATR"() -> (w1820:refnum<vi>)
            n715 = property class="Tbl (strict)"(reference=w1820, error in=w1808) -> ("Value"=w1821:string[][])  [unwired: 2 out]
            n716 = control-ref of="ATR"() -> (w1748:refnum<vi>)
            n717 = call "PassFailUUT (SubVI).vi"("Table in"=w1748) -> ("PassFaileUUTresult"=w1741:bool)  [unwired: 8 in, 2 out]
            n718 = property on="Test Failed" class="Bool (strict)"("Value"=w1741) -> ()  [unwired: 2 in, 2 out]
            n719 = property on="PN" class="Str"() -> ("Value"=w1731:string)  [unwired: 2 in, 2 out]
            n720 = call "MarvinReport.vi"("HEADER1"=w1756, "ATR Or"=w1820, "Steps   pfull"=w1821, "Footer UUT"=w1776, "pageNum"=3, "InputHeaderArray"=w1755, "FILE NAME"=w1799, "Report Folder"=w1797, "PN"=w1731, "REV"=w1784, "Test-Conductor"=w1761) -> ("error out"=w1771:errorcluster)  [unwired: 3 in, 1 out]
            n721 = Select(t="PASS" ("name or relative path"), s=w1741, f="FAIL" ("name or relative path")) -> (s? t:f=w1740:string)
            n722 = call <vilib>:"Clear Errors.vi"("error in (no error)"=w1771) -> ("error out"=w1770:errorcluster)  [unwired: 5 in, 1 out]
            n723 = property class="Bool (strict)"(reference=w1782, error in=w1770) -> ("BoolText.Text"=w1781:string)  [unwired: 2 out]
            n724 = Equal?(x=w1781, y="Report") -> (x = y?=w1775:bool)
            n725 = Select(t=T2."MainProgram", s=w1775, f=T2."MainProgram") -> (s? t:f=w1778:T2)
            n726 = call <vilib>:"Application Directory.vi"() -> ("Application Directory"=w1744:path)
            n727 = Build Path(base path=w1744, name or relative path="data\\TestResult.ini") -> (appended path=w1747:path)
            n728 = Select(t="Save Report...", s=w1775, f="Program Stopped...\r\nPlease turn OFF All Power sinks") -> (s? t:f=w1773:string)
            n729 = property on="Report" class="Bool (strict)"(error in=w1770, "Value"=w1732) -> (error out=w1733:errorcluster)  [unwired: 1 in, 1 out]
            n730 = call <vilib>:"Open Config Data.vi"("configuration file path"=w1747) -> ("error out"=w1745:errorcluster, "refnum"=w1746:T3)  [unwired: 2 in, 7 out]
            n731 = property on="Stop Button" class="Bool (strict)"(error in=w1733, "Value"=w1732) -> ()  [unwired: 1 in, 2 out]
            n732 = property on="Pannel User Message" class="Str"("Value"=w1773) -> ()  [unwired: 2 in, 2 out]
            n733 = call-poly <vilib>:"Write Key.vi"("section"="Kinetics", "error in (no error)"=w1745, "value"=w1740, "key"="Result", "refnum"=w1746) -> ("error out"=w1743:errorcluster, "refnum out"=w1742:T3)  [unwired: 4 in, 1 out]
            n734 = call <vilib>:"Close Config Data.vi"("error in (no error)"=w1743, "refnum"=w1742) -> ()  [unwired: 8 in, 2 out]
          }
          event "Help Button": Value Change {
            n735 = event-data() -> ()  [unwired: 1 in, 6 out]
            n736 = vi-ref "Help.vi"() -> (w1886:refnum<vi>)
            n737 = invoke class="VI" method="FP.Open"(reference=w1886, error in=w1884, "Activate"=TRUE ("Activate?"), "State"=T11."Standard") -> (error out=w1885:errorcluster)  [unwired: 1 in, 4 out]
            n738 = call "Help.vi"("error in"=w1885, "TesterSWVersion"=w1878) -> ("error out"=w1883:errorcluster)  [unwired: 6 in]
            n739 = property on="Help Button" class="Bool (strict)"("Value"=FALSE ("Help Button")) -> ()  [unwired: 2 in, 2 out]
          }
          event "Serial Com": Value Change {
            n740 = event-data() -> ()  [unwired: 1 in, 6 out]
            n741 = property on="Serial Com" class="Bool"(error in=w1895, "Visible"=FALSE) -> (error out=w1899:errorcluster)  [unwired: 1 in, 1 out]
            n742 = property on="VISA Kinetics" class="VISAName"(error in=w1899, "Visible"=TRUE) -> (error out=w1896:errorcluster)  [unwired: 1 in, 1 out]
          }
          event "VISA Kinetics": Value Change {
            n743 = event-data() -> ()  [unwired: 1 in, 6 out]
            n744 = property on="Serial Com" class="Bool"(error in=w1903, "Visible"=FALSE) -> ()  [unwired: 1 in, 2 out]
            n745 = property on="Pannel User Message" class="Str"(error in=w1903, "Value"="Serial connection in process" ("Pannel User Message")) -> ()  [unwired: 1 in, 2 out]
          }
          event "Refresh Button": Value Change {
            n746 = event-data() -> ()  [unwired: 1 in, 6 out]
          }
          event "Settings": Value Change {
            n747 = event-data() -> ()  [unwired: 1 in, 6 out]
          }
        }
      }
      frame "Initialize" {
        w1939 = 0
        w1942 = FALSE ("Visible")
        w1926 = refnum<visa-resource-name> "COMx" ("VISA resource name")
        w1934 = FALSE ("Serial Status")
        n748 = property on="EventTimeout" class="DigNum (strict)"(error in=errorcluster {"status"=FALSE, "code"=0, "source"=""} ("error out"), "Value"=100 ("EventTimeout")) -> (error out=w1937:errorcluster)  [unwired: 1 in, 1 out]
        n749 = property on="ComTestResult" class="Bool (strict)"("Value"=w1942) -> ()  [unwired: 2 in, 2 out]
        n750 = property on="VenableResult" class="Bool (strict)"("Value"=w1942) -> ()  [unwired: 2 in, 2 out]
        n751 = property on="VenableDirectionResult" class="Bool (strict)"("Value"=w1942) -> ()  [unwired: 2 in, 2 out]
        n752 = property on="Serial Com" class="Bool"(error in=w1937, "Visible"=FALSE) -> (error out=w1947:errorcluster)  [unwired: 1 in, 1 out]
        n753 = property on="VISA Kinetics" class="VISAName"(error in=w1947, "Visible"=FALSE, "Value"=w1926) -> (error out=w1938:errorcluster)  [unwired: 1 in, 1 out]
        n754 = property on="Refresh Button" class="Bool (strict)"(error in=w1938, "Value"=FALSE ("Refresh Button")) -> (error out=w1925:errorcluster)  [unwired: 1 in, 1 out]
        n755 = property on="Serial Status" class="Bool (strict)"("Value"=w1934) -> ()  [unwired: 2 in, 2 out]
        n756 = property on="Automation" class="Bool (strict)"("Value"=FALSE ("Visible")) -> ()  [unwired: 2 in, 2 out]
        n757 = disable-structure shown="Enabled" {
          disable-tunnel: w1926 -> [w1955 w1957]
          disable-tunnel: w1925 -> [w1954 w1958]
          disable-tunnel: [w1952 w1958] -> w1924
          disable-tunnel: [w1950 w1957] -> w1923
          disable-tunnel: [w1949 TRUE ("Tester Status")] -> w1922
          frame Disabled {
            n758 = call "COM Tester.vi"("error in (no error)"=w1954, "VISA resource name 2"=w1955) -> ("error out"=w1953:errorcluster, ".not. x?"=w1949:bool, "VISA Current"=w1950:refnum<visa-resource-name>)  [unwired: 7 in]
            n759 = call "RS232 DTR RTS.vi"("error in (no error)"=w1953, "Func"=enum16{"Init", "VEnable", "PowerOnOff"}."Init", "TesterCOM in"=w1950) -> ("error out"=w1952:errorcluster)  [unwired: 8 in]
          }
          frame Enabled {
          }
        }
        "TesterCOM" <- w1923
        "Tester Status" <- w1922
        n760 = call "COM Curent Read.vi"("error in (no error)"=w1924, "VISA resource name 2"=w1926) -> ("error out"=w1932:errorcluster, "VISA Current"=w1931:refnum<visa-resource-name>)  [unwired: 7 in, 1 out]
        "VISA Current" <- w1931
        n761 = call "ReadCurrent.vi"("error in (no error)"=w1932, "LoopFromMain"=TRUE, "VISA resource name"=w1931) -> ("error out"=w1929:errorcluster, "CurrentSens"=w1930:bool, "CurrentOut"=w1928:string)  [unwired: 6 in]
        n762 = property on="CurrentSens" class="Bool (strict)"("Value"=w1930) -> ()  [unwired: 2 in, 2 out]
        n763 = property on="Current" class="Str"("Value"=w1928) -> ()  [unwired: 2 in, 2 out]
        "Test Failed" <- w1934
      }
    }
  }
  n764 = call "ATRBuild.vi"() -> ()  [unwired: 9 in, 3 out]
  n765 = disable-structure shown="Disabled" {
    frame Disabled {
      n766 = case shown="\"BLDC 30A\", Default" {
        selector: _ -> [_ _ _ _ _]
        tunnel: [26 26 26 26 35] -> _
        frame "BLDC 30A", Default {
        }
        frame "Warrior 60A" {
        }
        frame "Condenser Merkava" {
        }
        frame "Condenser India" {
        }
        frame "BLDC 60A" {
        }
      }
    }
    frame Enabled {
    }
  }
  n767 = disable-structure shown="Disabled" {
    frame Disabled {
      n768 = control-ref of="Stop Button"() -> ()  [unwired: 1 out]
      n769 = control-ref of="UUT"() -> ()  [unwired: 1 out]
      n770 = property on="UUT" class="Str" props=["Value"]() -> ()  [unwired: 2 in, 3 out]
      n771 = control-ref of="UUT"() -> ()  [unwired: 1 out]
      n772 = property on="UUT" class="DigNum (strict)" props=["Value"]() -> ()  [unwired: 2 in, 3 out]
      n773 = control-ref of="Motor Speed RPM Serial"() -> ()  [unwired: 1 out]
      n774 = call "Find_Number_LineMARVIN.vi"() -> ()  [unwired: 5 in, 4 out]
      n775 = control-ref of="Pannel User Message"() -> ()  [unwired: 1 out]
      n776 = call "Write panel message Kinetics (SubVI).vi"() -> ()  [unwired: 10 in, 2 out]
      n777 = control-ref of="ATR"() -> ()  [unwired: 1 out]
      n778 = call "PassOrFail (SubVI).vi"() -> ()  [unwired: 11 in, 1 out]
      n779 = local read item#-1() -> (w1965)
      n780 = call "Serial.vi"("write buffer"="EP=1\r\nVC=1000\r\n") -> ()  [unwired: 9 in, 2 out]
      n781 = call "RS232 DTR RTS.vi"(7:w1965) -> ()  [unwired: 10 in, 1 out]
      n782 = property on="UUT" class="Str" props=["Value"]() -> ()  [unwired: 2 in, 3 out]
    }
    frame Enabled {
    }
  }
  n783 = disable-structure shown="Disabled" {
    frame Disabled {
      w1966 = T9."Disabled and Grayed Out" ("Disabled")
      w1967 = FALSE ("Start")
      n784 = property on="Current SN" class="DigNum (strict)" props=["Value"]() -> ()  [unwired: 2 in, 3 out]
      n785 = property on="UUT" class="DigNum (strict)" props=["Value"]() -> ()  [unwired: 2 in, 3 out]
      n786 = property on="Serial Status" class="Bool (strict)" props=["Value"]() -> ()  [unwired: 2 in, 3 out]
      n787 = property on="UUT SoftwareVer" class="Str" props=["Value"]() -> ()  [unwired: 2 in, 3 out]
      n788 = call "RS232 DTR RTS.vi"() -> ()  [unwired: 11 in, 1 out]
      n789 = property on="Next SN" class="DigNum (strict)" props=["Value"]() -> ()  [unwired: 3 in, 2 out]
      n790 = property on="Start" class="Bool (strict)"("Value"=w1967, "DisabledEnum"=w1966) -> ()  [unwired: 2 in, 2 out]
      n791 = property on="Report" class="Bool (strict)"("Value"=w1967, "DisabledEnum"=w1966) -> ()  [unwired: 2 in, 2 out]
    }
    frame Enabled {
    }
  }
  "Pannel User Message" <- w18
